vi "TestColletion2.vi"() -> ()   [LabVIEW 2018]
uses:
  <vilib>/Utility/error.llb/whitespace.ctl
panel:
  out "数据处理 2":bool
  out "AI0":bool
  out "AI1":bool
  out "AI2":bool
  out "AI3":bool
  out "AI4":bool
  out "AI5":bool
  out "AI6":bool
  out "AI7":bool
  out "AI8":bool
  out "AI9":bool
  out "AI10":bool
  out "AI11":bool
  out "AI12":bool
  out "AI13":bool
  out "AI14":bool
  out "AI15":bool
  out "数据处理及上传控制":i32
  out "数据1":dbl[](array[numeric])
  out "输出数组1":dbl[](array[numeric])
  out "AI 0 size(s)":i32
  out "数据2":dbl[](array[numeric])
  out "数据3":dbl[](array[numeric])
  out "数据4":dbl[](array[numeric])
  out "数据5":dbl[](array[numeric])
  out "数据6":dbl[](array[numeric])
  out "数据7":dbl[](array[numeric])
  out "数据8":dbl[](array[numeric])
  out "数据9":dbl[](array[numeric])
  out "数据10":dbl[](array[numeric])
  out "数据11":dbl[](array[numeric])
  out "数据12":dbl[](array[numeric])
  out "数据13":dbl[](array[numeric])
  out "数据14":dbl[](array[numeric])
  out "数据15":dbl[](array[numeric])
  out "数据16":dbl[](array[numeric])
  out "输出数组16":dbl[](array[numeric])
  out "输出数组15":dbl[](array[numeric])
  out "输出数组14":dbl[](array[numeric])
  out "输出数组13":dbl[](array[numeric])
  out "输出数组12":dbl[](array[numeric])
  out "输出数组11":dbl[](array[numeric])
  out "输出数组10":dbl[](array[numeric])
  out "输出数组9":dbl[](array[numeric])
  out "输出数组8":dbl[](array[numeric])
  out "输出数组7":dbl[](array[numeric])
  out "输出数组6":dbl[](array[numeric])
  out "输出数组5":dbl[](array[numeric])
  out "输出数组4":dbl[](array[numeric])
  out "输出数组3":dbl[](array[numeric])
  out "输出数组2":dbl[](array[numeric])
  out "大小":i32
  out "数组":string[][](array[string])
  out "数值 3":i32
  out "字符串":string
  out "数值 2":i32
  out "数值":i32
  out "特征值16":string
  out "特征值15":string
  out "特征值14":string
  out "特征值13":string
  out "特征值12":string
  out "特征值11":string
  out "特征值10":string
  out "特征值9":string
  out "特征值8":string
  out "特征值7":string
  out "特征值6":string
  out "特征值5":string
  out "特征值4":string
  out "特征值3":string
  out "特征值2":string
  out "特征值1":string
  in  "XB_NLP2.IClass1":refnum<k7>
  in  "noisy1.IClass1":refnum<k7>
  out "AI 1 size(s)":i32
  in  "输入电压":sgl(ring)=5.0 items=["10"=10, "5"=5]
  out "SQL语句":string
  in  "通道模式":u8(ring)=3 items=["DIFF"=0, "NRSE"=1, "RSE"=3]
  in  "驱动编号":i32
  out "subarray":string[](array[string])
  in  "停止":bool
  out "AI 15 size(s)":i32
  out "AI 14 size(s)":i32
  out "AI 13 size(s)":i32
  out "AI 12 size(s)":i32
  out "AI 11 size(s)":i32
  out "AI 10 size(s)":i32
  out "AI 9 size(s)":i32
  out "AI 8 size(s)":i32
  out "AI 7 size(s)":i32
  out "AI 4 size(s)":i32
  out "AI 5 size(s)":i32
  out "AI 6 size(s)":i32
  out "AI 3 size(s)":i32
  out "AI 2 size(s)":i32
  in  "主选项卡":T1(tab)
  in  "采样次数":u32=5 format="采样次数：%.0f"
  in  "搜索按钮":bool
  in  "间隔时间":i32 format="时间(min)：%.0f"
  in  "sym":string="sym10"
  in  "lev":i32=3 format="lev: %.0f"
  out "数据库状态":errorcluster caption="采集卡状态"
  out "采集卡状态":errorcluster
  in  "暂停":bool
  in  "关闭":bool
  in  "延时":bool
  out "布尔":bool
  in  "数据处理":bool
  in  "初始化":bool
  out "上传到数据库":bool
  in  "数据库":bool
  in  "开始":bool
  in  "主页按钮 8":bool
  in  "主页按钮 9":bool
  out "当前时间":timestamp format="时间：%<%H:%M:%S %x>T"
  in  "查看单传感器采集的数据":bool
  in  "历史查询":bool
  in  "查看当前特征值":bool
  in  "查看当前数据波形":bool
  in  "查看去噪后波形":bool
  in  "创建特征值数据表":bool
  in  "创建原始数据表":bool
  in  "通道选择":bool[](array[boolean])=[TRUE, FALSE, FALSE, FALSE, FALSE, FALSE, FALSE, FALSE, FALSE, FALSE, FALSE, FALSE, FALSE, FALSE, FALSE, FALSE]
  out "过程提示":string
  in  "采样率":u32=1000 format="采样率：%.0f"
  in  "主页按钮 2":bool
  in  "清空传感器数据表":bool
  in  "清空数据":bool
  in  "显示全部数据":bool
  in  "保存16个传感器的数据":bool
  out "全部数据":string[][](table)
  in  "主页按钮":bool
  in  "原始数据选项卡":enum32{"1 - 8", "9 - 16"}(tab)
  out "AI 3 波形":dbl[](graph)
  out "AI 2 波形":dbl[](graph)
  out "AI 1 波形":dbl[](graph)
  out "AI 4 波形":dbl[](graph)
  out "AI 5 波形":dbl[](graph)
  out "AI 7 波形":dbl[](graph)
  out "AI 6 波形":dbl[](graph)
  out "AI 11 波形":dbl[](graph)
  out "AI 8 波形":dbl[](graph)
  out "AI 9 波形":dbl[](graph)
  out "AI 10 波形":dbl[](graph)
  out "AI 12 波形":dbl[](graph)
  out "AI 13 波形":dbl[](graph)
  out "AI 14 波形":dbl[](graph)
  out "AI 15 波形":dbl[](graph)
  in  "主页按钮 3":bool
  in  "去噪波形选项卡":enum32{"1 - 8 ", "9 - 16"}(tab)
  out "AI2去噪后波形图":dbl[][](graph)
  out "AI3去噪后波形图":dbl[][](graph)
  out "AI4去噪后波形图":dbl[][](graph)
  out "AI5去噪后波形图":dbl[][](graph)
  out "AI6去噪后波形图":dbl[][](graph)
  out "AI7去噪后波形图":dbl[][](graph)
  out "AI1去噪后波形图":dbl[][](graph)
  out "AI0去噪后波形图":dbl[][](graph)
  out "AI8去噪后波形图":dbl[][](graph)
  out "AI9去噪后波形图":dbl[][](graph)
  out "AI10去噪后波形图":dbl[][](graph)
  out "AI11去噪后波形图":dbl[][](graph)
  out "AI2去噪后波形图":dbl[][](graph)
  out "AI13去噪后波形图":dbl[][](graph)
  out "AI14去噪后波形图":dbl[][](graph)
  out "AI15去噪后波形图":dbl[][](graph)
  in  "主页按钮 4":bool
  out "AI0特征值":dbl[][](array[numeric])
  out "AI1特征值":dbl[][](array[numeric])
  out "AI3特征值":dbl[][](array[numeric])
  out "AI5特征值":dbl[][](array[numeric])
  out "AI4特征值":dbl[][](array[numeric])
  out "AI2特征值":dbl[][](array[numeric])
  out "AI6特征值":dbl[][](array[numeric])
  out "AI8特征值":dbl[][](array[numeric])
  out "AI10特征值":dbl[][](array[numeric])
  out "AI11特征值":dbl[][](array[numeric])
  out "AI12特征值":dbl[][](array[numeric])
  out "AI13特征值":dbl[][](array[numeric])
  out "AI14特征值":dbl[][](array[numeric])
  out "AI7特征值":dbl[][](array[numeric])
  out "AI9特征值":dbl[][](array[numeric])
  out "AI15特征值":dbl[][](array[numeric])
  in  "主页按钮 5":bool
  in  "历史查询选项卡":enum32{"原始数据查询", "健康值查询"}(tab)
  out "状态提示":string
  out "波形图 2":dbl[](graph)
  out "查询数据":string[][](table)
  in  "文件名":string
  in  "保存地址":path
  in  "保存":bool
  in  "传感器":T2(ring)
  in  "查询":bool
  in  "从":timestamp
  in  "到":timestamp
  in  "传感器":T2(ring)
  in  "到":timestamp
  in  "从":timestamp
  out "健康值查询结果":string[][](table)
  in  "显示健康值":bool
  in  "传感器数据查询":bool
  in  "健康值查询":bool
  in  "主页按钮 6":bool
  out "波形图 3":dbl[](graph)
  out "当前组波形":dbl[](graph)
  in  "主页按钮 7":bool
  out "AI0特征值 2":dbl[][](array[numeric])
  out "去噪后波形图":dbl[][](graph)
  # "包装设备状态监测与预测系统"
  # "请务必将传感器接到采集卡的 AI 0 通道"
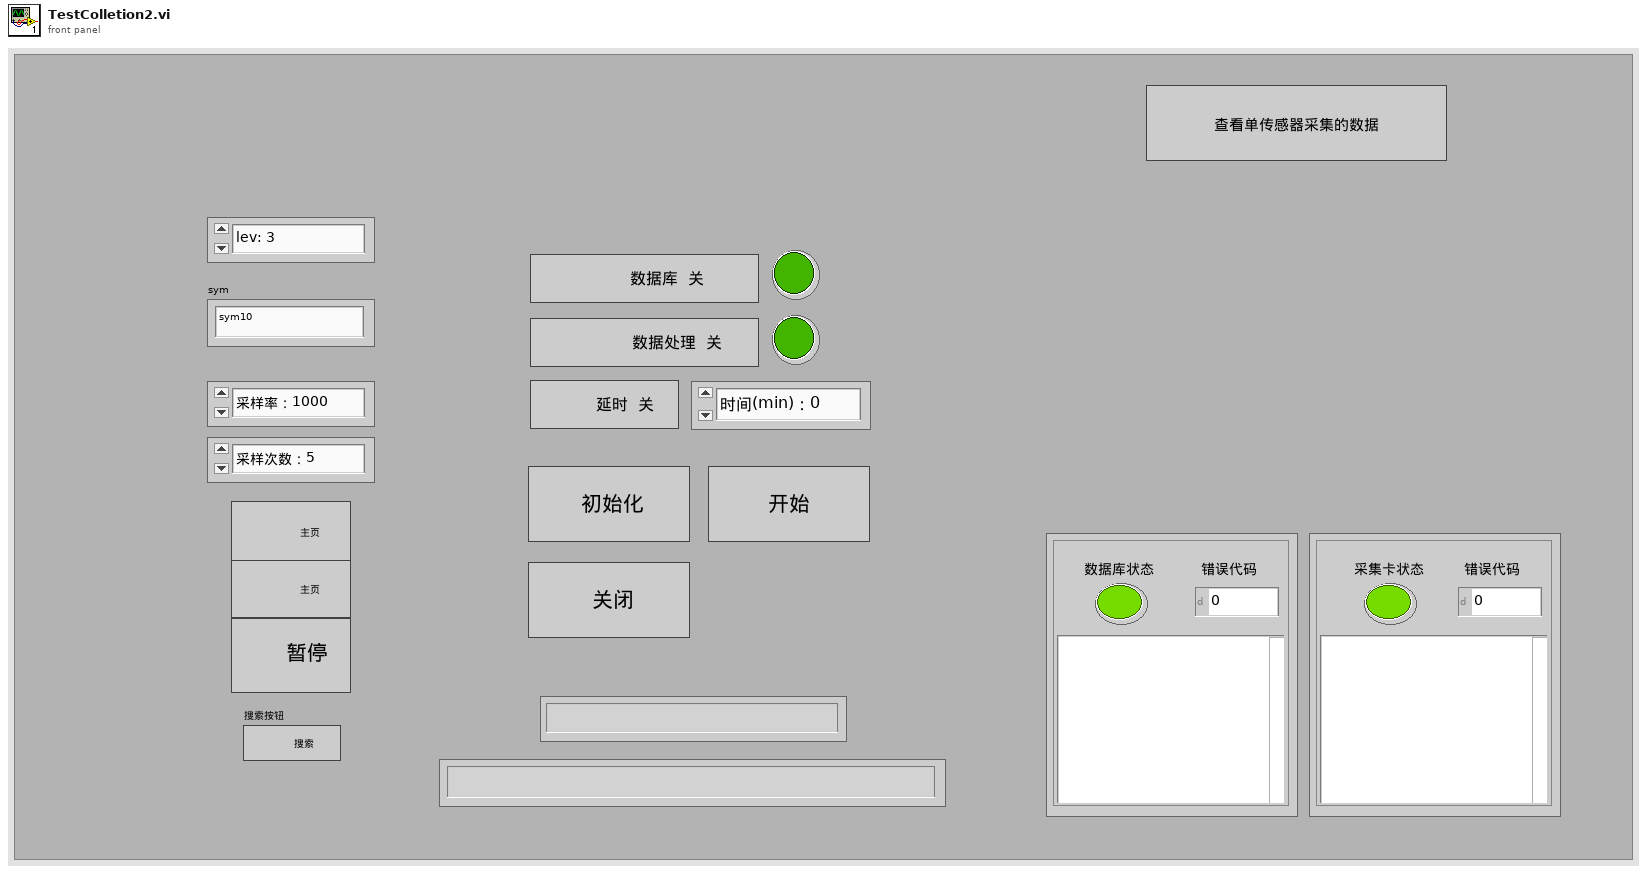
[diagram p1: front panel]
types:
  T1 = enum32{"端口设置", "传感器数据", "原始数据波形", "去噪后的波形", "特征值数据", "健康值记录", "历史查询", "单传感器测试"}
  T2 = enum16{"sensor1", "sensor2", "sensor3", "sensor4", "sensor5", "sensor6", "sensor7", "sensor8", "sensor9", "sensor10", "sensor11", "sensor12", "sensor13", "sensor14", "sensor15", "sensor16"}
  T3 = typedef "whitespace.ctl" = u16
  T4 = enum16{"open", "replace", "create", "open or create", "replace or create", "replace or create with confirmation"}
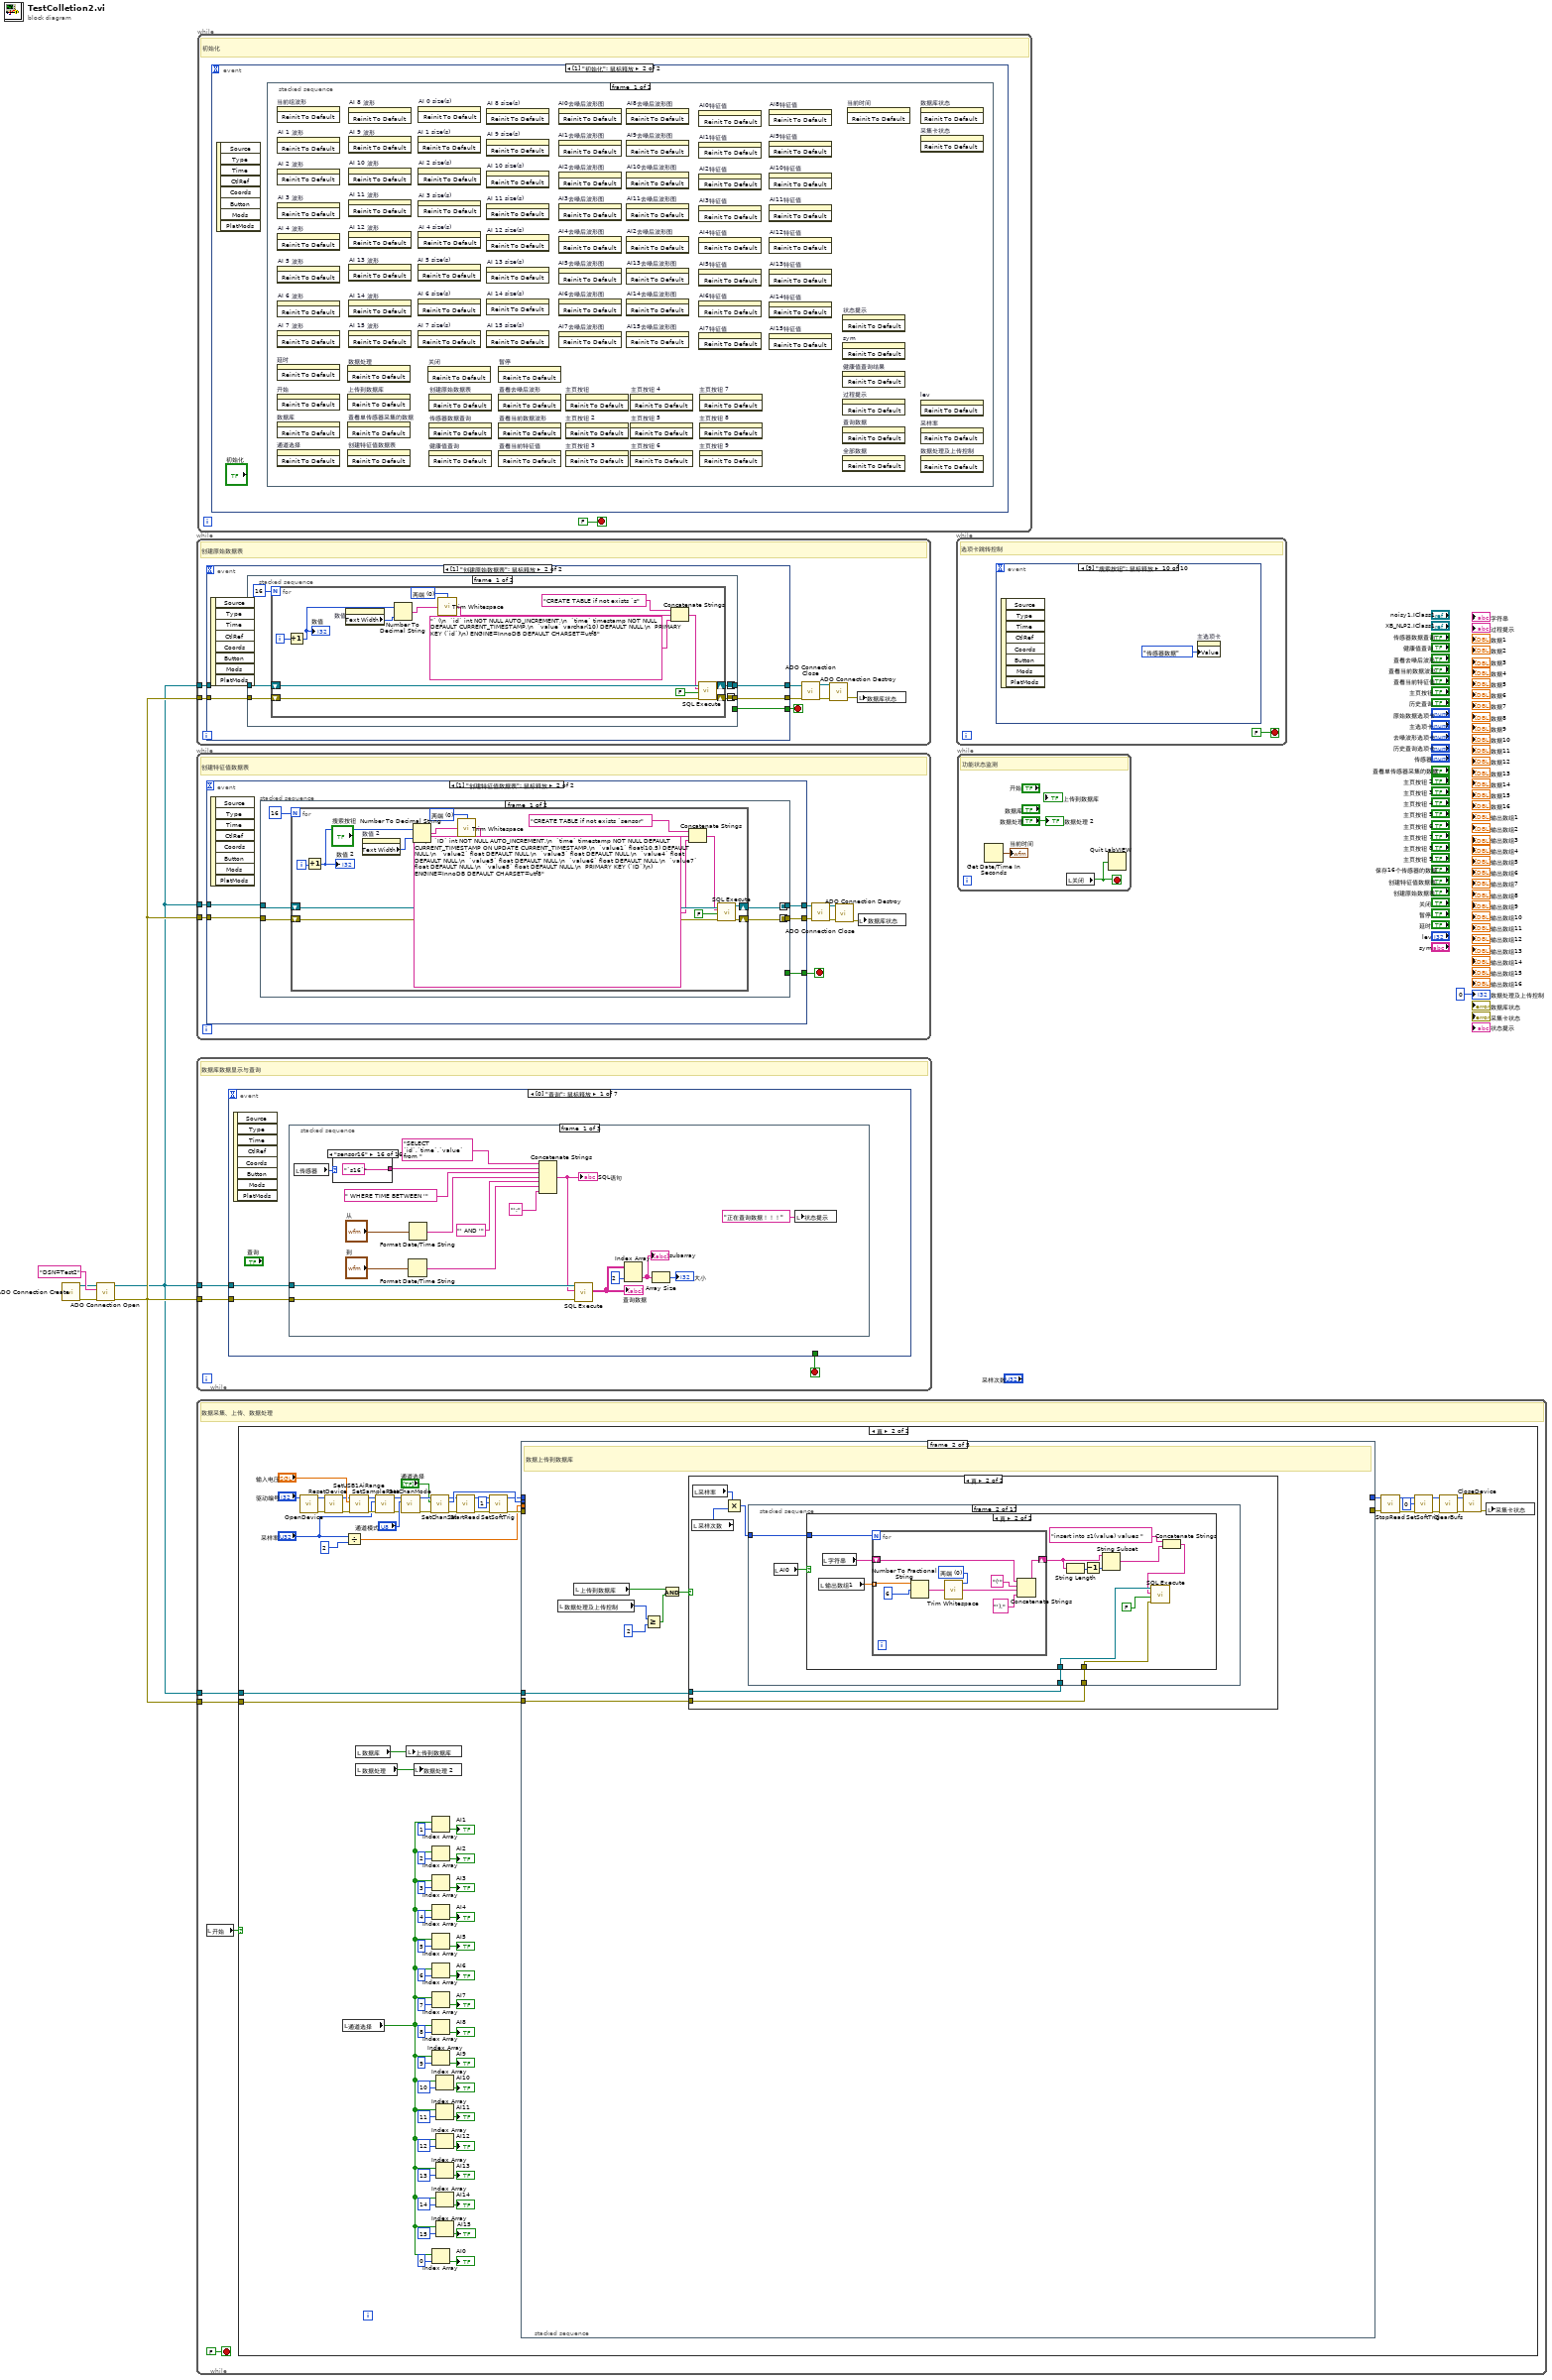
[diagram p0: block diagram]
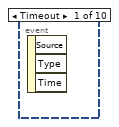
[diagram p2: hidden frame]
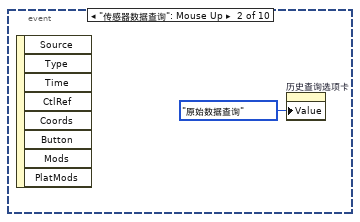
[diagram p3: hidden frame]
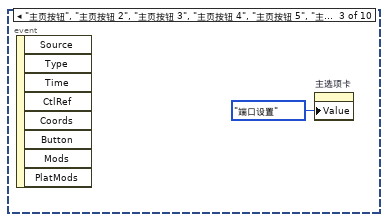
[diagram p4: hidden frame]
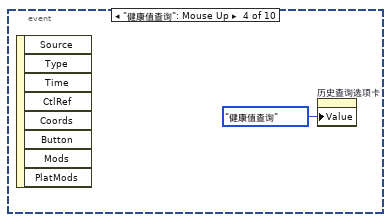
[diagram p5: hidden frame]
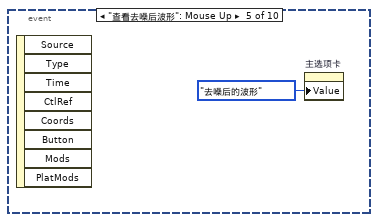
[diagram p6: hidden frame]
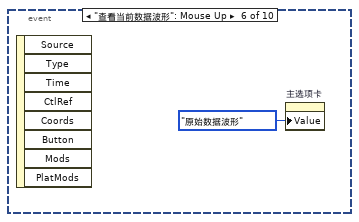
[diagram p7: hidden frame]
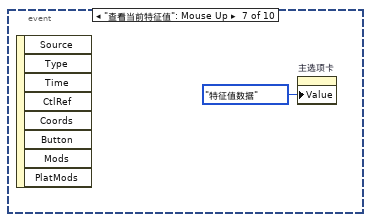
[diagram p8: hidden frame]
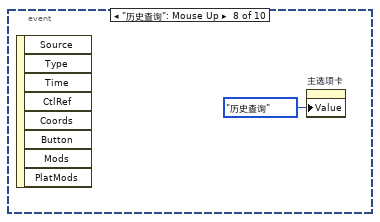
[diagram p9: hidden frame]
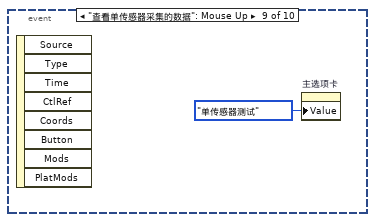
[diagram p10: hidden frame]
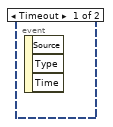
[diagram p11: hidden frame]
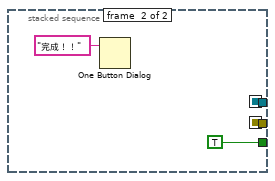
[diagram p12: hidden frame]
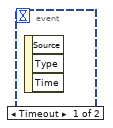
[diagram p13: hidden frame]
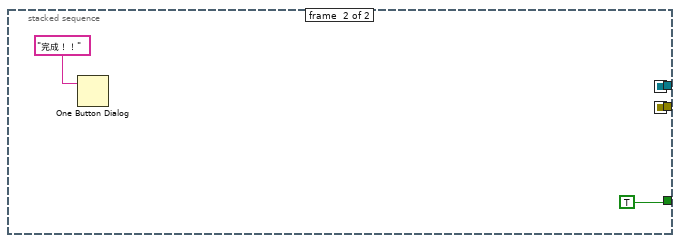
[diagram p14: hidden frame]
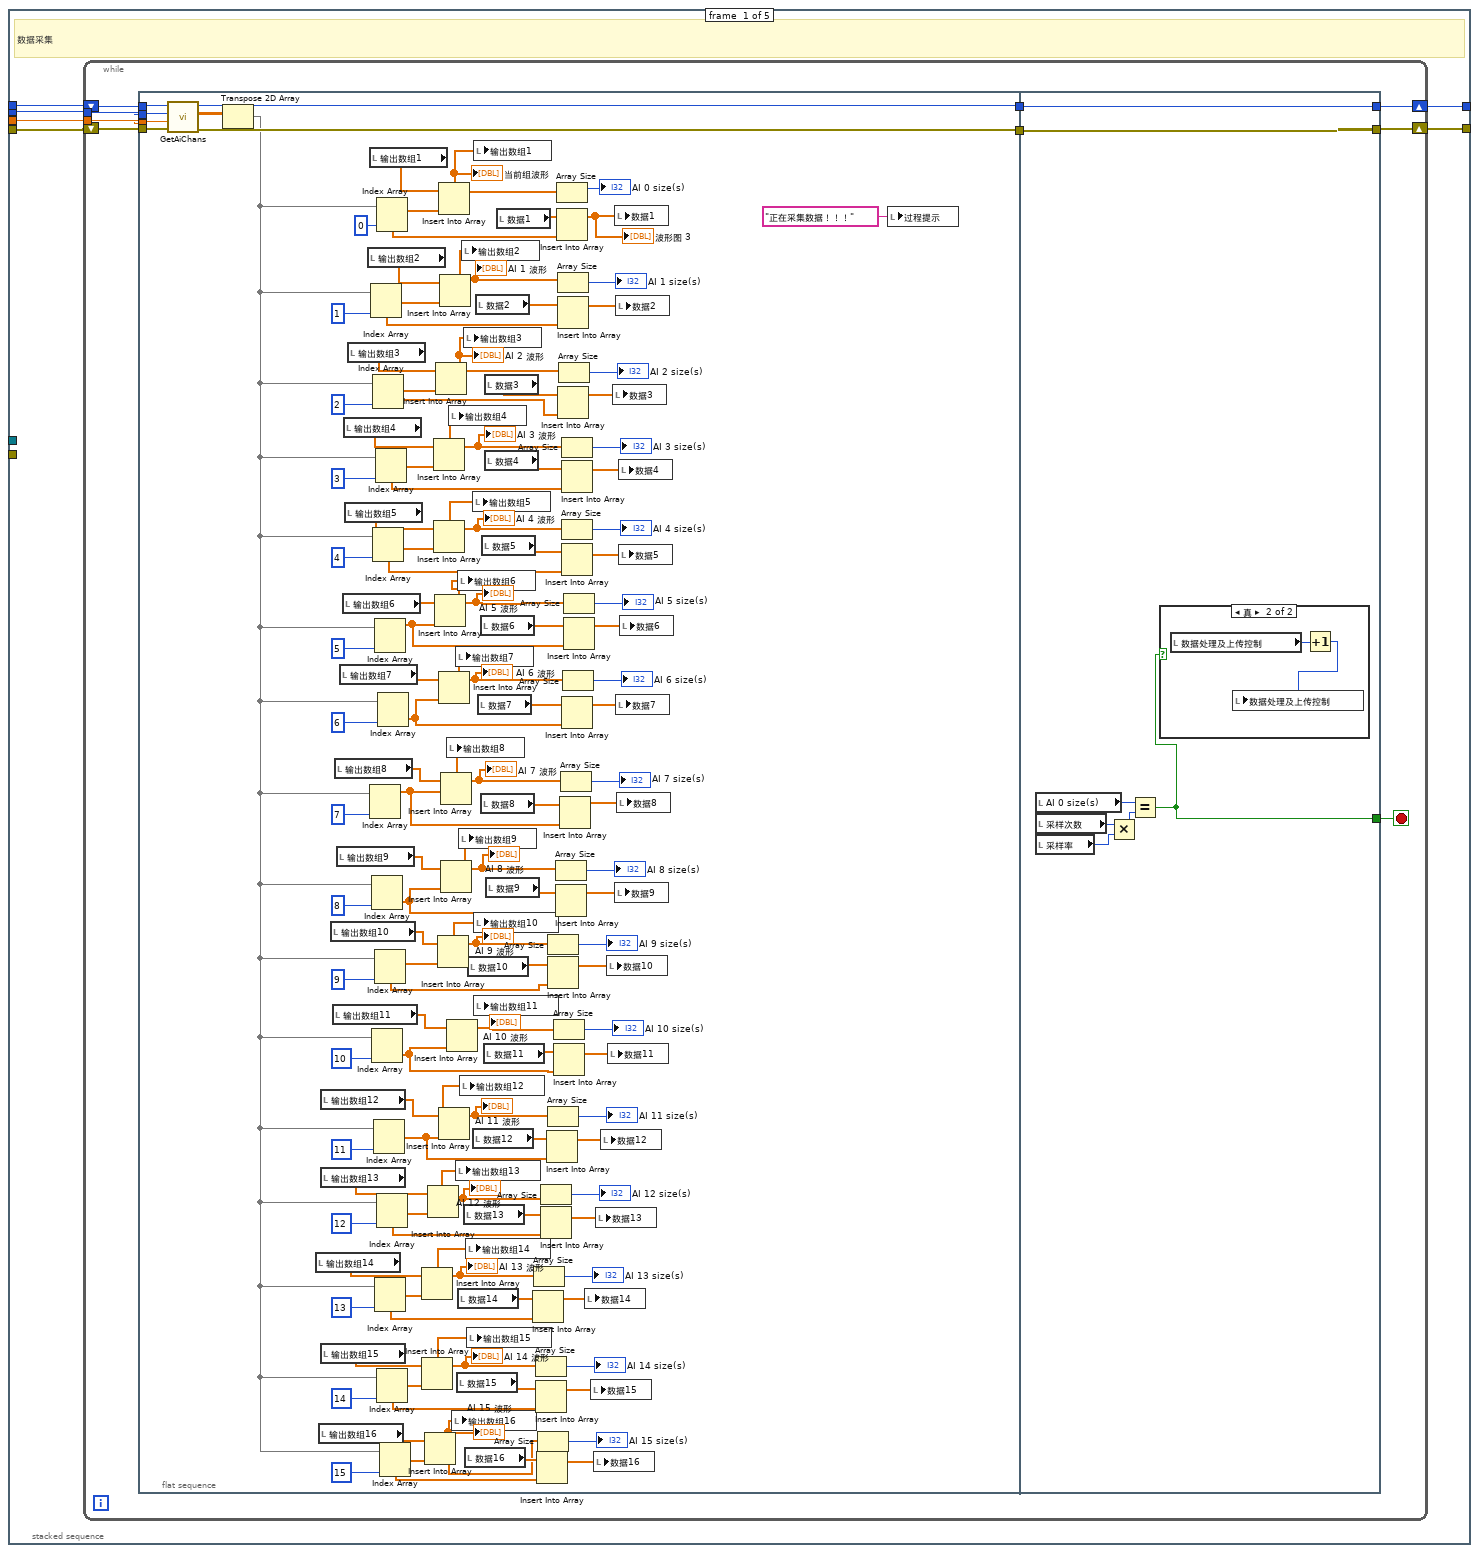
[diagram p16: hidden frame]
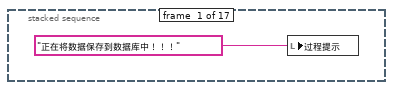
[diagram p19: hidden frame]
diagram:
  n1 = call "ADO Connection Create.vi"() -> ("error out"=w4:errorcluster, "ADODB._Connection Out"=w5:refnum<k7>)  [unwired: 10 in]
  n2 = call "ADO Connection Open.vi"("error in (no error)"=w4, "ConnectionString"="DSN=Test2", "ADODB._Connection In"=w5) -> ("error out"=w3:errorcluster, "ADODB._Connection Out"=w2:refnum<k7>)  [unwired: 7 in]
  n3 = while {
    tunnel: w3 -> [w14]
    tunnel: w2 -> [w13]
    stop <- w8 stop-if-true
    # "创建原始数据表"
    n4 = event shown="[1] \"创建原始数据表\": 鼠标释放" {
      selector: _ -> [_ _]
      dyn-events: _ -> [_ _]
      timeout: _ -> [_ _]
      tunnel: w13 -> [_ w19]
      tunnel: w14 -> [_ w18]
      tunnel: [_ w17] -> w9
      tunnel: [_ w16] -> w10
      tunnel: [_ w15] -> w8
      event Timeout {
        n5 = event-data() -> ()  [unwired: 1 in, 3 out]
      }
      event "创建原始数据表": Mouse Up {
        n6 = event-data() -> ()  [unwired: 1 in, 8 out]
        n7 = stacked-sequence {
          seq-local: [w22 _] -> [_ w42]
          seq-local: [w21 _] -> [_ w41]
          tunnel: w19 -> [w24 _]
          tunnel: w18 -> [w23 _]
          tunnel: [_ w42] -> w17
          tunnel: [_ w41] -> w16
          tunnel: [_ TRUE] -> w15
          frame #0 {
            n8 = for {
              N: 16 -> [_]
              shift-right: [w34] -> w21
              shift-left: w24 -> [w38]
              shift-right: [w35] -> w22
              shift-left: w23 -> [w37]
              i -> [w26]
              w28 = T3 0 items=["两端", "字符串首端", "字符串末端"] ("location (both)")
              n9 = Increment(x=w26) -> (x+1=w25:i32)
              "数值" <- w25
              n10 = property on="数值" class="DigNum (严格)"() -> ("Text Width"=w27:u32)  [unwired: 2 in, 2 out]
              n11 = Number To Decimal String(number=w25, width (-)=w27) -> (decimal integer string=w30:string)
              n12 = call <vilib>:"Trim Whitespace.vi"("string"=w30, "location (both)"=w28) -> ("trimmed string"=w29:string)
              n13 = Concatenate Strings("CREATE TABLE if not exists `s", w29, "` (\n  `id` int NOT NULL AUTO_INCREMENT,\n  `time` timestamp NOT NULL DEFAULT CURRENT_TIMESTAMP,\n  `value` varchar(10) DEFAULT NULL,\n  PRIMARY KEY (`id`)\n) ENGINE=InnoDB DEFAULT CHARSET=utf8") -> (w31:string)
              n14 = call "SQL Execute.vi"("error in (no error)"=w37, "Return Data (T)"=FALSE, "Command Text"=w31, "ADODB._Connection In"=w38) -> ("error out"=w35:errorcluster, "ADODB._Connection Out"=w34:refnum<k7>)  [unwired: 4 in, 2 out]
            }
          }
          frame #1 {
            n15 = One Button Dialog(message="完成！！" ("消息")) -> ()  [unwired: 1 in, 1 out]
          }
        }
      }
    }
    n16 = call "ADO Connection Close.vi"("error in (no error)"=w9, "ADODB._Connection In"=w10) -> ("error out"=w11:errorcluster, "ADODB._Connection Out"=w12:refnum<k7>)  [unwired: 8 in]
    n17 = call "ADO Connection Destroy.vi"("error in (no error)"=w11, "ADODB._Connection In"=w12) -> ("error out"=w7:errorcluster)  [unwired: 9 in]
    n18 = local write "数据库状态"(w7) -> ()
  }
  n19 = while {
    tunnel: w3 -> [w50]
    tunnel: w2 -> [w49]
    stop <- w44 stop-if-true
    # "创建特征值数据表"
    n20 = event shown="[1] \"创建特征值数据表\": 鼠标释放" {
      selector: _ -> [_ _]
      dyn-events: _ -> [_ _]
      timeout: _ -> [_ _]
      tunnel: w49 -> [_ w55]
      tunnel: w50 -> [_ w54]
      tunnel: [_ w53] -> w45
      tunnel: [_ w52] -> w46
      tunnel: [_ w51] -> w44
      event Timeout {
        n21 = event-data() -> ()  [unwired: 1 in, 3 out]
      }
      event "创建特征值数据表": Mouse Up {
        n22 = event-data() -> ()  [unwired: 1 in, 8 out]
        n23 = stacked-sequence {
          seq-local: [w57 _] -> [_ w78]
          seq-local: [w56 _] -> [_ w77]
          tunnel: w55 -> [w59 _]
          tunnel: w54 -> [w58 _]
          tunnel: [_ w78] -> w53
          tunnel: [_ w77] -> w52
          tunnel: [_ TRUE] -> w51
          frame #0 {
            n24 = for {
              N: 16 -> [_]
              shift-right: [w70] -> w57
              shift-left: w59 -> [w74]
              shift-right: [w71] -> w56
              shift-left: w58 -> [w73]
              i -> [w62]
              w64 = T3 0 items=["两端", "字符串首端", "字符串末端"] ("location (both)")
              n25 = Increment(x=w62) -> (x+1=w61:i32)
              "数值 2" <- w61
              n26 = property on="数值 2" class="DigNum (严格)"() -> ("Text Width"=w63:u32)  [unwired: 2 in, 2 out]
              n27 = Number To Decimal String(number=w61, width (-)=w63) -> (decimal integer string=w66:string)
              n28 = call <vilib>:"Trim Whitespace.vi"("string"=w66, "location (both)"=w64) -> ("trimmed string"=w65:string)
              n29 = Concatenate Strings("CREATE TABLE if not exists `sensor", w65, "` (\n  `ID` int NOT NULL AUTO_INCREMENT,\n  `time` timestamp NOT NULL DEFAULT CURRENT_TIMESTAMP ON UPDATE CURRENT_TIMESTAMP,\n  `value1` float(10,5) DEFAULT NULL,\n  `value2` float DEFAULT NULL,\n  `value3` float DEFAULT NULL,\n  `value4` float DEFAULT NULL,\n  `value5` float DEFAULT NULL,\n  `value6` float DEFAULT NULL,\n  `value7` float DEFAULT NULL,\n  `value8` float DEFAULT NULL,\n  PRIMARY KEY (`ID`)\n) ENGINE=InnoDB DEFAULT CHARSET=utf8") -> (w67:string)
              n30 = call "SQL Execute.vi"("error in (no error)"=w73, "Return Data (T)"=FALSE, "Command Text"=w67, "ADODB._Connection In"=w74) -> ("error out"=w71:errorcluster, "ADODB._Connection Out"=w70:refnum<k7>)  [unwired: 4 in, 2 out]
            }
          }
          frame #1 {
            n31 = One Button Dialog(message="完成！！" ("消息")) -> ()  [unwired: 1 in, 1 out]
          }
        }
      }
    }
    n32 = call "ADO Connection Close.vi"("error in (no error)"=w46, "ADODB._Connection In"=w45) -> ("error out"=w47:errorcluster, "ADODB._Connection Out"=w48:refnum<k7>)  [unwired: 8 in]
    n33 = call "ADO Connection Destroy.vi"("error in (no error)"=w47, "ADODB._Connection In"=w48) -> ("error out"=w43:errorcluster)  [unwired: 9 in]
    n34 = local write "数据库状态"(w43) -> ()
  }
  n35 = while {
    tunnel: w3 -> [w81]
    tunnel: w2 -> [w80]
    stop <- w79 stop-if-true
    # "数据库数据显示与查询"
    n36 = event shown="[0] \"查询\": 鼠标释放" {
      selector: _ -> [_ _ _ _ _ _ _]
      dyn-events: _ -> [_ _ _ _ _ _ _]
      timeout: _ -> [_ _ _ _ _ _ _]
      tunnel: w81 -> [w82 _ _ w151 w172 w191 _]
      tunnel: w80 -> [w83 _ _ w152 w173 w190 _]
      tunnel: [_ _ TRUE _ _ _ _] -> w79
      event "查询": Mouse Up {
        n37 = event-data() -> ()  [unwired: 1 in, 8 out]
        n38 = stacked-sequence {
          tunnel: w83 -> [w101 _ _]
          tunnel: w82 -> [w100 _ _]
          frame #0 {
            n39 = local read "传感器"() -> (w91:T2)
            n40 = case shown="\"sensor16\"" w91 {
              tunnel: ["`s1`" "`s2`" "`s3`" "`s4`" "`s5`" "`s6`" "`s7`" "`s8`" "`s9`" "`s10`" "`s11`" "`s12`" "`s13`" "`s14`" "`s15`" "`s16`"] -> w86
              frame "sensor1", Default {
              }
              frame "sensor2" {
              }
              frame "sensor3" {
              }
              frame "sensor4" {
              }
              frame "sensor5" {
              }
              frame "sensor6" {
              }
              frame "sensor7" {
              }
              frame "sensor8" {
              }
              frame "sensor9" {
              }
              frame "sensor10" {
              }
              frame "sensor11" {
              }
              frame "sensor12" {
              }
              frame "sensor13" {
              }
              frame "sensor14" {
              }
              frame "sensor15" {
              }
              frame "sensor16" {
              }
            }
            n41 = Format Date/Time String(seconds (now)="到") -> (date/time string=w94:string)  [unwired: 2 in]
            n42 = Format Date/Time String(seconds (now)="从") -> (date/time string=w93:string)  [unwired: 2 in]
            n43 = Concatenate Strings("SELECT `id`,`time`,`value` from " ("string"), w86, " WHERE TIME BETWEEN '" ("string"), w93, "' AND '" ("string"), w94, "';" ("string")) -> (w97:string)
            "SQL语句" <- w97
            n44 = call "SQL Execute.vi"("error in (no error)"=w100, "Command Text"=w97, "ADODB._Connection In"=w101) -> ("Data"=w88:string[][])  [unwired: 5 in, 3 out]
            "查询数据" <- w88
            n45 = Index Array(array=w88, index (col)=2 ("disabled index (col)")) -> (element=w89:string[])  [unwired: 1 in]
            "subarray" <- w89
            n46 = Array Size(array=w89) -> (size(s)=→"大小":i32)
            n47 = local write "状态提示"("正在查询数据！！！" ("状态提示")) -> ()
          }
          frame #1 {
            n48 = local read "大小"() -> (w120:i32)
            n49 = for {
              N: w120 -> [_]
              shift-right: [w122] -> w119
              shift-left: dbl[] [] -> [w123]
              i -> [w125]
              n50 = local read "subarray"() -> (w126:string[])
              n51 = Index Array(array=w126, index=w125) -> (element=w128:string)
              n52 = Fract/Exp String To Number(string=w128) -> (number=w127:dbl)  [unwired: 3 in, 1 out]
              n53 = Build Array(w127) -> (w124:dbl[])
              n54 = Insert Into Array(array=w123, index=w125, new element=w124) -> (w122:dbl[])
            }
            "波形图 2" <- w119
            n55 = local write "状态提示"("正在绘制波形" ("状态提示")) -> ()
          }
          frame #2 {
            n56 = One Button Dialog(message="查询及绘图完成！！！" ("消息")) -> ()  [unwired: 1 in, 1 out]
          }
        }
      }
      event "保存": Mouse Up {
        n57 = event-data() -> ()  [unwired: 1 in, 8 out]
        n58 = flat-sequence {
          frame #0 {
            n59 = property on="查询数据" class="Tbl (严格)"() -> ("Value"=w137:string[][])  [unwired: 2 in, 2 out]
            n60 = Index Array(array=w137, index (col)=2 ("disabled index (col)")) -> (element=w135:string[])  [unwired: 1 in]
            n61 = Concatenate Strings("文件名", ".csv" ("name or relative path")) -> (w141:string)
            n62 = Build Path(base path="保存地址", name or relative path=w141) -> (appended path=w142:path)
            n63 = Array To Spreadsheet String(delimiter (Tab)="\r\n", array=w135, 3:"" ("format string")) -> (spreadsheet string=w132:string)
            n64 = Open/Create/Replace File(file path (use dialog)=w142, operation (0:open)=T4."replace or create", access (0:read/write)=enum16{"read/write", "read-only", "write-only"}."read/write") -> (refnum out=w146:refnum<file>, error out=w147:errorcluster)  [unwired: 3 in, 1 out]
            n65 = Write to Binary File(file (use dialog)=w146, data=w132, error in=w147) -> (refnum out=w144:refnum<file>, error out=w145:errorcluster)  [unwired: 3 in, 1 out]
            n66 = Close File(refnum=w144, error in=w145) -> (error out=w143:errorcluster)  [unwired: 1 out]
            n67 = call <vilib>:"Simple Error Handler.vi"("error in (no error)"=w143) -> ()  [unwired: 4 in, 5 out]
          }
          frame #1 {
            n68 = One Button Dialog(message="数据保存完成！！！" ("消息")) -> ()  [unwired: 1 in, 1 out]
          }
        }
      }
      event "停止": Mouse Up {
        n69 = event-data() -> ()  [unwired: 1 in, 8 out]
      }
      event "显示全部数据": Mouse Up {
        n70 = event-data() -> ()  [unwired: 1 in, 8 out]
        n71 = for {
          N: 16 -> [_]
          tunnel: w152 -> [w169]
          tunnel: w151 -> [w168]
          i -> [w154]
          w162 = T3 0 items=["两端", "字符串首端", "字符串末端"] ("location (both)")
          n72 = Increment(x=w154) -> (x+1=w153:i32)
          "数值 3" <- w153
          n73 = property on="数值 3" class="DigNum (严格)"() -> ("Text Width"=w165:u32)  [unwired: 2 in, 2 out]
          n74 = Number To Fractional String(number=w153, width (-)=w165) -> (F-format string=w163:string)  [unwired: 2 in]
          n75 = call <vilib>:"Trim Whitespace.vi"("string"=w163, "location (both)"=w162) -> ("trimmed string"=w161:string)
          n76 = Concatenate Strings("select `value` from `s;" ("string"), w161, "`;") -> (w159:string)
          n77 = call "SQL Execute.vi"("error in (no error)"=w168, "Return Data (T)"=FALSE, "Command Text"=w159, "ADODB._Connection In"=w169) -> ("Data"=w167:string[][])  [unwired: 4 in, 3 out]
          n78 = Index Array(array=w167, index (col)=0 ("禁用的索引 (列)")) -> (element=w157:string[])  [unwired: 1 in]
          n79 = local read "数组"() -> (w158:string[][])
          n80 = Insert Into Array(array=w158, index (row)=w153, new element=w157) -> (→"全部数据":string[][])  [unwired: 1 in]
        }
      }
      event "显示健康值": Mouse Up {
        n81 = event-data() -> ()  [unwired: 1 in, 8 out]
        n82 = case shown="\"sensor16\"" "传感器" {
          tunnel: ["`s1`" "`s2`" "`s3`" "`s4`" "`s5`" "`s6`" "`s7`" "`s8`" "`s9`" "`s10`" "`s11`" "`s12`" "`s13`" "`s14`" "`s15`" "`s16`"] -> _
          frame "sensor1", Default {
          }
          frame "sensor2" {
          }
          frame "sensor3" {
          }
          frame "sensor4" {
          }
          frame "sensor5" {
          }
          frame "sensor6" {
          }
          frame "sensor7" {
          }
          frame "sensor8" {
          }
          frame "sensor9" {
          }
          frame "sensor10" {
          }
          frame "sensor11" {
          }
          frame "sensor12" {
          }
          frame "sensor13" {
          }
          frame "sensor14" {
          }
          frame "sensor15" {
          }
          frame "sensor16" {
          }
        }
        n83 = call "SQL Execute.vi"("error in (no error)"=w172, "Command Text"="", "ADODB._Connection In"=w173) -> ()  [unwired: 5 in, 4 out]
      }
      event "清空数据": Mouse Up {
        # "清空数据库的全部数据"
        n84 = event-data() -> ()  [unwired: 1 in, 8 out]
        n85 = call "SQL Execute.vi"("error in (no error)"=w191, "Return Data (T)"=FALSE, "Command Text"="truncate s1;" ("string"), "ADODB._Connection In"=w190) -> ()  [unwired: 4 in, 4 out]
        n86 = One Button Dialog(message="数据已全部清除", button name ("OK")="确定     ") -> ()  [unwired: 1 out]
      }
      event "清空传感器数据表": Mouse Up {
        n87 = event-data() -> ()  [unwired: 1 in, 8 out]
        n88 = flat-sequence {
          frame #0 {
            n89 = invoke on="全部数据" class="Tbl (strict)" method="Reinit To Default"() -> ()  [unwired: 3 in, 3 out]
          }
          frame #1 {
            n90 = One Button Dialog(message="清空完毕！！！" ("消息")) -> ()  [unwired: 1 in, 1 out]
          }
        }
      }
    }
  }
  n91 = while {
    tunnel: w3 -> [w197]
    tunnel: w2 -> [w198]
    stop <- FALSE stop-if-true
    # "数据采集、上传、数据处理"
    n92 = local read "开始"() -> (w199:bool)
    n93 = case shown="真" w199 {
      tunnel: w198 -> [_ w262]
      tunnel: w197 -> [_ w261]
      frame False {
      }
      frame True {
        n94 = call "OpenDevice.vi"("DevIndex"="驱动编号") -> ("错误输出"=w244:errorcluster, "DevIndex Output"=w245:i32)  [unwired: 9 in]
        n95 = call "ResetDevice.vi"("错误输入（无错误）"=w244, "DevIndex"=w245) -> ("错误输出"=w247:errorcluster, "DevIndex Output"=w248:i32)  [unwired: 8 in]
        n96 = local read "通道选择"() -> (w203:bool[])
        n97 = Divide(x="采样率", y=u32 2) -> (x/y=w207:dbl)
        n98 = call "SetUSB1AiRange.vi"("错误输入（无错误）"=w247, "Range"="输入电压", "DevIndex"=w248) -> ("错误输出"=w250:errorcluster, "DevIndex Output"=w251:i32)  [unwired: 7 in]
        n99 = local read "数据库"() -> (w205:bool)
        n100 = local read "数据处理"() -> (w206:bool)
        n101 = call "SetSampleRate.vi"("错误输入（无错误）"=w250, "SampleRate"="采样率", "DevIndex"=w251) -> ("错误输出"=w252:errorcluster, "DevIndex Output"=w253:i32)  [unwired: 7 in]
        n102 = call "SetChanMode.vi"("错误输入（无错误）"=w252, "ChanMode"="通道模式", "DevIndex"=w253) -> ("错误输出"=w255:errorcluster, "DevIndex Output"=w256:i32)  [unwired: 7 in]
        n103 = local write "上传到数据库"(w205) -> ()
        n104 = local write "数据处理 2"(w206) -> ()
        n105 = call "SetChanSel.vi"("错误输入（无错误）"=w255, "ChanSel"="通道选择", "DevIndex"=w256) -> ("错误输出"=w260:errorcluster, "ChanSel"=w264:u16, "DevIndex Output"=w259:i32)  [unwired: 6 in]
        n106 = Index Array(array=w203, index=1) -> (element=→"AI1":bool)
        n107 = Index Array(array=w203, index=2) -> (element=→"AI2":bool)
        n108 = Index Array(array=w203, index=3) -> (element=→"AI3":bool)
        n109 = Index Array(array=w203, index=4) -> (element=→"AI4":bool)
        n110 = Index Array(array=w203, index=5) -> (element=→"AI5":bool)
        n111 = Index Array(array=w203, index=6) -> (element=→"AI6":bool)
        n112 = Index Array(array=w203, index=7) -> (element=→"AI7":bool)
        n113 = Index Array(array=w203, index=8) -> (element=→"AI8":bool)
        n114 = Index Array(array=w203, index=9) -> (element=→"AI9":bool)
        n115 = Index Array(array=w203, index=0) -> (element=→"AI0":bool)
        n116 = Index Array(array=w203, index=10) -> (element=→"AI10":bool)
        n117 = Index Array(array=w203, index=11) -> (element=→"AI11":bool)
        n118 = Index Array(array=w203, index=12) -> (element=→"AI12":bool)
        n119 = Index Array(array=w203, index=13) -> (element=→"AI13":bool)
        n120 = Index Array(array=w203, index=14) -> (element=→"AI14":bool)
        n121 = Index Array(array=w203, index=15) -> (element=→"AI15":bool)
        n122 = call "StartRead.vi"("错误输入（无错误）"=w260, "DevIndex"=w259) -> ("错误输出"=w257:errorcluster, "DevIndex Output"=w258:i32)  [unwired: 8 in]
        n123 = call "SetSoftTrig.vi"("错误输入（无错误）"=w257, "Trig"=u8 1, "DevIndex"=w258) -> ("错误输出"=w265:errorcluster, "DevIndex Output"=w263:i32)  [unwired: 7 in]
        n124 = stacked-sequence {
          tunnel: w262 -> [_ w424 w837 _ _]
          tunnel: w261 -> [_ w423 w836 _ _]
          tunnel: w265 -> [w275 _ _ _ _]
          tunnel: w207 -> [w276 _ _ _ _]
          tunnel: w264 -> [w277 _ _ _ _]
          tunnel: w263 -> [w278 _ _ _ _]
          tunnel: [w274 _ _ _ _] -> w242
          tunnel: [w273 _ _ _ _] -> w241
          frame #0 {
            # "数据采集"
            n125 = while {
              tunnel: w277 -> [w286]
              tunnel: w276 -> [w280]
              shift-right: [w285] -> w274
              shift-left: w278 -> [w287]
              shift-right: [w284] -> w273
              shift-left: w275 -> [w279]
              stop <- w281 stop-if-true
              n126 = flat-sequence {
                tunnel: w287 -> [w361]
                tunnel: w286 -> [w360]
                tunnel: w280 -> [w359]
                tunnel: w279 -> [w357]
                tunnel: [w356] -> w283
                tunnel: [w355] -> w282
                tunnel: [w414] -> w284
                tunnel: [w415] -> w285
                tunnel: w283 -> [w415]
                tunnel: w282 -> [w414]
                tunnel: [w412] -> w281
                frame #0 {
                  n127 = call "GetAiChans.vi"("错误输入（无错误）"=w357, "Num"=w359, "ChanSel"=w360, "DevIndex"=w361) -> ("错误输出"=w355:errorcluster, "Ai"=w358:sgl[][], "DevIndex Output"=w356:i32)  [unwired: 4 in, 1 out]
                  n128 = Transpose 2D Array(2D array=w358) -> (transposed array=w288:sgl[][])
                  n129 = local read "输出数组14"() -> (w364:dbl[])
                  n130 = local read "输出数组16"() -> (w362:dbl[])
                  n131 = local read "输出数组12"() -> (w366:dbl[])
                  n132 = local read "输出数组13"() -> (w365:dbl[])
                  n133 = local read "输出数组15"() -> (w363:dbl[])
                  n134 = local read "输出数组10"() -> (w368:dbl[])
                  n135 = local read "输出数组11"() -> (w367:dbl[])
                  n136 = local read "输出数组8"() -> (w370:dbl[])
                  n137 = local read "输出数组9"() -> (w369:dbl[])
                  n138 = local read "输出数组7"() -> (w371:dbl[])
                  n139 = local read "输出数组6"() -> (w372:dbl[])
                  n140 = local read "输出数组4"() -> (w374:dbl[])
                  n141 = local read "输出数组5"() -> (w373:dbl[])
                  n142 = local read "输出数组3"() -> (w375:dbl[])
                  n143 = local read "输出数组2"() -> (w376:dbl[])
                  n144 = local read "输出数组1"() -> (w377:dbl[])
                  n145 = Index Array(array=w288, index (col)=7 ("disabled index (col)")) -> (element=w334:sgl[])  [unwired: 1 in]
                  n146 = Index Array(array=w288, index (col)=1 ("disabled index (col)")) -> (element=w352:sgl[])  [unwired: 1 in]
                  n147 = Index Array(array=w288, index (col)=8 ("disabled index (col)")) -> (element=w331:sgl[])  [unwired: 1 in]
                  n148 = Index Array(array=w288, index (col)=10 ("disabled index (col)")) -> (element=w325:sgl[])  [unwired: 1 in]
                  n149 = Index Array(array=w288, index (col)=2 ("disabled index (col)")) -> (element=w349:sgl[])  [unwired: 1 in]
                  n150 = Index Array(array=w288, index (col)=4 ("disabled index (col)")) -> (element=w343:sgl[])  [unwired: 1 in]
                  n151 = Index Array(array=w288, index (col)=11 ("disabled index (col)")) -> (element=w322:sgl[])  [unwired: 1 in]
                  n152 = Index Array(array=w288, index (col)=5 ("disabled index (col)")) -> (element=w340:sgl[])  [unwired: 1 in]
                  n153 = Index Array(array=w288, index (col)=9 ("disabled index (col)")) -> (element=w328:sgl[])  [unwired: 1 in]
                  n154 = Index Array(array=w288, index (col)=13 ("disabled index (col)")) -> (element=w315:sgl[])  [unwired: 1 in]
                  n155 = Index Array(array=w288, index (col)=3 ("disabled index (col)")) -> (element=w346:sgl[])  [unwired: 1 in]
                  n156 = Index Array(array=w288, index (col)=0 ("index (row)")) -> (element=w354:sgl[])  [unwired: 1 in]
                  n157 = Index Array(array=w288, index (col)=12 ("disabled index (col)")) -> (element=w319:sgl[])  [unwired: 1 in]
                  n158 = Index Array(array=w288, index (col)=14 ("disabled index (col)")) -> (element=w313:sgl[])  [unwired: 1 in]
                  n159 = Index Array(array=w288, index (col)=6 ("disabled index (col)")) -> (element=w337:sgl[])  [unwired: 1 in]
                  n160 = Index Array(array=w288, index (col)=15 ("disabled index (col)")) -> (element=w309:sgl[])  [unwired: 1 in]
                  n161 = Insert Into Array(array=w364, new element=w315) -> (w291:dbl[])  [unwired: 1 in]
                  "AI 13 波形" <- w291
                  n162 = Insert Into Array(array=w363, new element=w313) -> (w290:dbl[])  [unwired: 1 in]
                  "AI 14 波形" <- w290
                  n163 = Insert Into Array(array=w362, new element=w309) -> (w289:dbl[])  [unwired: 1 in]
                  "AI 15 波形" <- w289
                  n164 = Insert Into Array(array=w365, new element=w319) -> (w292:dbl[])  [unwired: 1 in]
                  "AI 12 波形" <- w292
                  n165 = Insert Into Array(array=w374, new element=w346) -> (w301:dbl[])  [unwired: 1 in]
                  "AI 3 波形" <- w301
                  n166 = Insert Into Array(array=w373, new element=w343) -> (w300:dbl[])  [unwired: 1 in]
                  "AI 4 波形" <- w300
                  n167 = Insert Into Array(array=w372, new element=w340) -> (w299:dbl[])  [unwired: 1 in]
                  "AI 5 波形" <- w299
                  n168 = Insert Into Array(array=w375, new element=w349) -> (w302:dbl[])  [unwired: 1 in]
                  "AI 2 波形" <- w302
                  n169 = Insert Into Array(array=w368, new element=w328) -> (w295:dbl[])  [unwired: 1 in]
                  "AI 9 波形" <- w295
                  n170 = Insert Into Array(array=w377, new element=w354) -> (w306:dbl[])  [unwired: 1 in]
                  "当前组波形" <- w306
                  n171 = Insert Into Array(array=w371, new element=w337) -> (w297:dbl[])  [unwired: 1 in]
                  "AI 6 波形" <- w297
                  n172 = Insert Into Array(array=w366, new element=w322) -> (w293:dbl[])  [unwired: 1 in]
                  "AI 11 波形" <- w293
                  n173 = Insert Into Array(array=w376, new element=w352) -> (w303:dbl[])  [unwired: 1 in]
                  "AI 1 波形" <- w303
                  n174 = Insert Into Array(array=w370, new element=w334) -> (w298:dbl[])  [unwired: 1 in]
                  "AI 7 波形" <- w298
                  n175 = Insert Into Array(array=w369, new element=w331) -> (w296:dbl[])  [unwired: 1 in]
                  "AI 8 波形" <- w296
                  n176 = local write "输出数组8"(w298) -> ()
                  n177 = Insert Into Array(array=w367, new element=w325) -> (w294:dbl[])  [unwired: 1 in]
                  "AI 10 波形" <- w294
                  n178 = local write "输出数组4"(w301) -> ()
                  n179 = local write "输出数组16"(w289) -> ()
                  n180 = local write "输出数组7"(w297) -> ()
                  n181 = local write "输出数组13"(w292) -> ()
                  n182 = local read "数据15"() -> (w312:dbl[])
                  n183 = local write "输出数组6"(w299) -> ()
                  n184 = local read "数据14"() -> (w316:dbl[])
                  n185 = local write "输出数组9"(w296) -> ()
                  n186 = local write "输出数组12"(w293) -> ()
                  n187 = local write "输出数组2"(w303) -> ()
                  n188 = local write "输出数组3"(w302) -> ()
                  n189 = local read "数据13"() -> (w318:dbl[])
                  n190 = local read "数据16"() -> (w310:dbl[])
                  n191 = local write "输出数组14"(w291) -> ()
                  n192 = local write "输出数组15"(w290) -> ()
                  n193 = local read "数据10"() -> (w327:dbl[])
                  n194 = local write "输出数组5"(w300) -> ()
                  n195 = local read "数据12"() -> (w321:dbl[])
                  n196 = local write "输出数组1"(w306) -> ()
                  n197 = local write "输出数组10"(w295) -> ()
                  n198 = local write "输出数组11"(w294) -> ()
                  n199 = local read "数据2"() -> (w351:dbl[])
                  n200 = local read "数据7"() -> (w336:dbl[])
                  n201 = local read "数据6"() -> (w339:dbl[])
                  n202 = local read "数据8"() -> (w333:dbl[])
                  n203 = local read "数据5"() -> (w342:dbl[])
                  n204 = local read "数据11"() -> (w324:dbl[])
                  n205 = local read "数据3"() -> (w348:dbl[])
                  n206 = local read "数据4"() -> (w345:dbl[])
                  n207 = local read "数据9"() -> (w330:dbl[])
                  n208 = local read "数据1"() -> (w353:dbl[])
                  n209 = Insert Into Array(array=w316, new element=w315) -> (w314:dbl[])  [unwired: 1 in]
                  n210 = Array Size(array=w291) -> (size(s)=→"AI 13 size(s)":i32)
                  n211 = Array Size(array=w290) -> (size(s)=→"AI 14 size(s)":i32)
                  n212 = Insert Into Array(array=w312, new element=w313) -> (w311:dbl[])  [unwired: 1 in]
                  n213 = Insert Into Array(array=w310, new element=w309) -> (w308:dbl[])  [unwired: 1 in]
                  n214 = Array Size(array=w289) -> (size(s)=→"AI 15 size(s)":i32)
                  n215 = Array Size(array=w292) -> (size(s)=→"AI 12 size(s)":i32)
                  n216 = Insert Into Array(array=w318, new element=w319) -> (w317:dbl[])  [unwired: 1 in]
                  n217 = Insert Into Array(array=w321, new element=w322) -> (w320:dbl[])  [unwired: 1 in]
                  n218 = Array Size(array=w295) -> (size(s)=→"AI 9 size(s)":i32)
                  n219 = Insert Into Array(array=w327, new element=w328) -> (w326:dbl[])  [unwired: 1 in]
                  n220 = Array Size(array=w293) -> (size(s)=→"AI 11 size(s)":i32)
                  n221 = Array Size(array=w294) -> (size(s)=→"AI 10 size(s)":i32)
                  n222 = Insert Into Array(array=w324, new element=w325) -> (w323:dbl[])  [unwired: 1 in]
                  n223 = Array Size(array=w296) -> (size(s)=→"AI 8 size(s)":i32)
                  n224 = Insert Into Array(array=w330, new element=w331) -> (w329:dbl[])  [unwired: 1 in]
                  n225 = Array Size(array=w306) -> (size(s)=→"AI 0 size(s)":i32)
                  n226 = Insert Into Array(array=w353, new element=w354) -> (w305:dbl[])  [unwired: 1 in]
                  "波形图 3" <- w305
                  n227 = Array Size(array=w303) -> (size(s)=→"AI 1 size(s)":i32)
                  n228 = Insert Into Array(array=w351, new element=w352) -> (w350:dbl[])  [unwired: 1 in]
                  n229 = Insert Into Array(array=w348, new element=w349) -> (w347:dbl[])  [unwired: 1 in]
                  n230 = Array Size(array=w302) -> (size(s)=→"AI 2 size(s)":i32)
                  n231 = Insert Into Array(array=w333, new element=w334) -> (w332:dbl[])  [unwired: 1 in]
                  n232 = Array Size(array=w298) -> (size(s)=→"AI 7 size(s)":i32)
                  n233 = Array Size(array=w301) -> (size(s)=→"AI 3 size(s)":i32)
                  n234 = Insert Into Array(array=w345, new element=w346) -> (w344:dbl[])  [unwired: 1 in]
                  n235 = Array Size(array=w300) -> (size(s)=→"AI 4 size(s)":i32)
                  n236 = Insert Into Array(array=w342, new element=w343) -> (w341:dbl[])  [unwired: 1 in]
                  n237 = Insert Into Array(array=w336, new element=w337) -> (w335:dbl[])  [unwired: 1 in]
                  n238 = Array Size(array=w297) -> (size(s)=→"AI 6 size(s)":i32)
                  n239 = Array Size(array=w299) -> (size(s)=→"AI 5 size(s)":i32)
                  n240 = Insert Into Array(array=w339, new element=w340) -> (w338:dbl[])  [unwired: 1 in]
                  n241 = local write "数据14"(w314) -> ()
                  n242 = local write "数据15"(w311) -> ()
                  n243 = local write "数据16"(w308) -> ()
                  n244 = local write "数据13"(w317) -> ()
                  n245 = local write "数据12"(w320) -> ()
                  n246 = local write "数据10"(w326) -> ()
                  n247 = local write "数据11"(w323) -> ()
                  n248 = local write "数据3"(w347) -> ()
                  n249 = local write "数据1"(w305) -> ()
                  n250 = local write "数据9"(w329) -> ()
                  n251 = local write "数据2"(w350) -> ()
                  n252 = local write "数据7"(w335) -> ()
                  n253 = local write "数据8"(w332) -> ()
                  n254 = local write "数据4"(w344) -> ()
                  n255 = local write "数据5"(w341) -> ()
                  n256 = local write "数据6"(w338) -> ()
                  n257 = local write "过程提示"("正在采集数据！！！" ("过程提示")) -> ()
                }
                frame #1 {
                  n258 = local read "AI 0 size(s)"() -> (w413:i32)
                  n259 = local read "采样次数"() -> (w411:u32)
                  n260 = local read "采样率"() -> (w410:u32)
                  n261 = Multiply(x=w411, y=w410) -> (x*y=w409:u32)
                  n262 = Equal?(x=w413, y=w409) -> (x = y?=w412:bool)
                  n263 = case shown="真" w412 {
                    frame False {
                    }
                    frame True {
                      n264 = local read "数据处理及上传控制"() -> (w417:i32)
                      n265 = Increment(x=w417) -> (x+1=w416:i32)
                      n266 = local write "数据处理及上传控制"(w416) -> ()
                    }
                  }
                }
              }
            }
          }
          frame #1 {
            # "数据上传到数据库"
            n267 = local read "数据处理及上传控制"() -> (w421:i32)
            n268 = local read "上传到数据库"() -> (w422:bool)
            n269 = Greater Or Equal?(x=w421, y=2) -> (x >= y?=w419:bool)
            n270 = And(x=w422, y=w419) -> (x .and. y?=w418:bool)
            n271 = case shown="真" w418 {
              tunnel: w424 -> [_ w428]
              tunnel: w423 -> [_ w429]
              frame False {
              }
              frame True {
                n272 = local read "采样次数"() -> (w426:u32)
                n273 = local read "采样率"() -> (w425:u32)
                n274 = Multiply(x=w425, y=w426) -> (x*y=w427:u32)
                n275 = stacked-sequence {
                  tunnel: w429 -> [_ w433 w459 w483 w508 w533 w558 w583 w608 w633 w658 w683 w708 w733 w758 w783 w808]
                  tunnel: w428 -> [_ w434 w458 w484 w509 w534 w559 w584 w609 w634 w659 w684 w709 w734 w759 w784 w809]
                  tunnel: w427 -> [_ w431 w456 w481 w506 w531 w556 w581 w606 w631 w656 w681 w706 w731 w756 w781 w806]
                  frame #0 {
                    n276 = local write "过程提示"("正在将数据保存到数据库中！！！" ("过程提示")) -> ()
                  }
                  frame #1 {
                    n277 = local read "AI0"() -> (w432:bool)
                    n278 = case shown="真" w432 {
                      tunnel: w434 -> [_ w444]
                      tunnel: w433 -> [_ w446]
                      tunnel: w431 -> [_ w435]
                      frame False {
                      }
                      frame True {
                        n279 = local read "输出数组1"() -> (w436:dbl[])
                        n280 = local read "字符串"() -> (w443:string)
                        n281 = for {
                          N: w435 -> [_]
                          tunnel: w436 -> [w452] mode=indexing
                          shift-right: [w450] -> w442
                          shift-left: w443 -> [w449]
                          w451 = T3 0 items=["两端", "字符串首端", "字符串末端"] ("location (both)")
                          n282 = Number To Fractional String(number=w452, width (-)=i16 6 ("宽度(-)")) -> (F-format string=w455:string)  [unwired: 2 in]
                          n283 = call <vilib>:"Trim Whitespace.vi"("string"=w455, "location (both)"=w451) -> ("trimmed string"=w453:string)
                          n284 = Concatenate Strings(w449, "('", w453, "')," ("字符串")) -> (w450:string)
                        }
                        n285 = String Length(string=w442) -> (length=w438:i32)
                        n286 = Decrement(x=w438) -> (x-1=w437:i32)
                        n287 = String Subset(string=w442, length (rest)=w437) -> (substring=w440:string)  [unwired: 1 in]
                        n288 = Concatenate Strings("insert into s1(value) values ", w440) -> (w439:string)
                        n289 = call "SQL Execute.vi"("error in (no error)"=w446, "Return Data (T)"=FALSE, "Command Text"=w439, "ADODB._Connection In"=w444) -> ()  [unwired: 4 in, 4 out]
                      }
                    }
                  }
                  frame #2 {
                    n290 = local read "AI1"() -> (w457:bool)
                    n291 = case shown="真" w457 {
                      tunnel: w459 -> [_ w465]
                      tunnel: w458 -> [_ w466]
                      tunnel: w456 -> [_ w460]
                      frame False {
                      }
                      frame True {
                        n292 = local read "字符串"() -> (w464:string)
                        n293 = local read "输出数组2"() -> (w461:dbl[])
                        n294 = for {
                          N: w460 -> [_]
                          shift-right: [w476] -> w470
                          shift-left: w464 -> [w475]
                          tunnel: w461 -> [w472] mode=indexing
                          w477 = T3 0 items=["两端", "字符串首端", "字符串末端"] ("location (both)")
                          n295 = Number To Fractional String(number=w472, width (-)=i16 6 ("宽度(-)")) -> (F-format string=w480:string)  [unwired: 2 in]
                          n296 = call <vilib>:"Trim Whitespace.vi"("string"=w480, "location (both)"=w477) -> ("trimmed string"=w478:string)
                          n297 = Concatenate Strings(w475, "('", w478, "')," ("字符串")) -> (w476:string)
                        }
                        n298 = String Length(string=w470) -> (length=w463:i32)
                        n299 = Decrement(x=w463) -> (x-1=w462:i32)
                        n300 = String Subset(string=w470, length (rest)=w462) -> (substring=w468:string)  [unwired: 1 in]
                        n301 = Concatenate Strings("insert into s2 (value) values ", w468) -> (w467:string)
                        n302 = call "SQL Execute.vi"("error in (no error)"=w465, "Return Data (T)"=FALSE, "Command Text"=w467, "ADODB._Connection In"=w466) -> ()  [unwired: 4 in, 4 out]
                      }
                    }
                  }
                  frame #3 {
                    n303 = local read "AI2"() -> (w482:bool)
                    n304 = case shown="真" w482 {
                      tunnel: w484 -> [_ w491]
                      tunnel: w483 -> [_ w490]
                      tunnel: w481 -> [_ w485]
                      frame False {
                      }
                      frame True {
                        n305 = local read "输出数组3"() -> (w486:dbl[])
                        n306 = local read "字符串"() -> (w489:string)
                        n307 = for {
                          N: w485 -> [_]
                          shift-right: [w501] -> w495
                          shift-left: w489 -> [w500]
                          tunnel: w486 -> [w497] mode=indexing
                          w502 = T3 0 items=["两端", "字符串首端", "字符串末端"] ("location (both)")
                          n308 = Number To Fractional String(number=w497, width (-)=i16 6 ("宽度(-)")) -> (F-format string=w505:string)  [unwired: 2 in]
                          n309 = call <vilib>:"Trim Whitespace.vi"("string"=w505, "location (both)"=w502) -> ("trimmed string"=w503:string)
                          n310 = Concatenate Strings(w500, "('", w503, "')," ("字符串")) -> (w501:string)
                        }
                        n311 = String Length(string=w495) -> (length=w488:i32)
                        n312 = Decrement(x=w488) -> (x-1=w487:i32)
                        n313 = String Subset(string=w495, length (rest)=w487) -> (substring=w493:string)  [unwired: 1 in]
                        n314 = Concatenate Strings("insert into s3 (value) values ", w493) -> (w492:string)
                        n315 = call "SQL Execute.vi"("error in (no error)"=w490, "Return Data (T)"=FALSE, "Command Text"=w492, "ADODB._Connection In"=w491) -> ()  [unwired: 4 in, 4 out]
                      }
                    }
                  }
                  frame #4 {
                    n316 = local read "AI3"() -> (w507:bool)
                    n317 = case shown="真" w507 {
                      tunnel: w509 -> [_ w516]
                      tunnel: w508 -> [_ w515]
                      tunnel: w506 -> [_ w510]
                      frame False {
                      }
                      frame True {
                        n318 = local read "输出数组4"() -> (w511:dbl[])
                        n319 = local read "字符串"() -> (w514:string)
                        n320 = for {
                          N: w510 -> [_]
                          shift-right: [w526] -> w520
                          shift-left: w514 -> [w525]
                          tunnel: w511 -> [w522] mode=indexing
                          w527 = T3 0 items=["两端", "字符串首端", "字符串末端"] ("location (both)")
                          n321 = Number To Fractional String(number=w522, width (-)=i16 6 ("宽度(-)")) -> (F-format string=w530:string)  [unwired: 2 in]
                          n322 = call <vilib>:"Trim Whitespace.vi"("string"=w530, "location (both)"=w527) -> ("trimmed string"=w528:string)
                          n323 = Concatenate Strings(w525, "('", w528, "')," ("字符串")) -> (w526:string)
                        }
                        n324 = String Length(string=w520) -> (length=w513:i32)
                        n325 = Decrement(x=w513) -> (x-1=w512:i32)
                        n326 = String Subset(string=w520, length (rest)=w512) -> (substring=w518:string)  [unwired: 1 in]
                        n327 = Concatenate Strings("insert into s4(value) values ", w518) -> (w517:string)
                        n328 = call "SQL Execute.vi"("error in (no error)"=w515, "Return Data (T)"=FALSE, "Command Text"=w517, "ADODB._Connection In"=w516) -> ()  [unwired: 4 in, 4 out]
                      }
                    }
                  }
                  frame #5 {
                    n329 = local read "AI4"() -> (w532:bool)
                    n330 = case shown="真" w532 {
                      tunnel: w534 -> [_ w540]
                      tunnel: w533 -> [_ w539]
                      tunnel: w531 -> [_ w535]
                      frame False {
                      }
                      frame True {
                        n331 = local read "输出数组5"() -> (w541:dbl[])
                        n332 = local read "字符串"() -> (w538:string)
                        n333 = for {
                          N: w535 -> [_]
                          shift-right: [w551] -> w545
                          shift-left: w538 -> [w550]
                          tunnel: w541 -> [w547] mode=indexing
                          w552 = T3 0 items=["两端", "字符串首端", "字符串末端"] ("location (both)")
                          n334 = Number To Fractional String(number=w547, width (-)=i16 6 ("宽度(-)")) -> (F-format string=w555:string)  [unwired: 2 in]
                          n335 = call <vilib>:"Trim Whitespace.vi"("string"=w555, "location (both)"=w552) -> ("trimmed string"=w553:string)
                          n336 = Concatenate Strings(w550, "('", w553, "')," ("字符串")) -> (w551:string)
                        }
                        n337 = String Length(string=w545) -> (length=w536:i32)
                        n338 = Decrement(x=w536) -> (x-1=w537:i32)
                        n339 = String Subset(string=w545, length (rest)=w537) -> (substring=w543:string)  [unwired: 1 in]
                        n340 = Concatenate Strings("insert into s5(value) values ", w543) -> (w542:string)
                        n341 = call "SQL Execute.vi"("error in (no error)"=w539, "Return Data (T)"=FALSE, "Command Text"=w542, "ADODB._Connection In"=w540) -> ()  [unwired: 4 in, 4 out]
                      }
                    }
                  }
                  frame #6 {
                    n342 = local read "AI5"() -> (w557:bool)
                    n343 = case shown="真" w557 {
                      tunnel: w559 -> [_ w565]
                      tunnel: w558 -> [_ w564]
                      tunnel: w556 -> [_ w560]
                      frame False {
                      }
                      frame True {
                        n344 = local read "字符串"() -> (w566:string)
                        n345 = local read "输出数组6"() -> (w561:dbl[])
                        n346 = for {
                          N: w560 -> [_]
                          shift-right: [w576] -> w570
                          shift-left: w566 -> [w575]
                          tunnel: w561 -> [w572] mode=indexing
                          w577 = T3 0 items=["两端", "字符串首端", "字符串末端"] ("location (both)")
                          n347 = Number To Fractional String(number=w572, width (-)=i16 6 ("宽度(-)")) -> (F-format string=w580:string)  [unwired: 2 in]
                          n348 = call <vilib>:"Trim Whitespace.vi"("string"=w580, "location (both)"=w577) -> ("trimmed string"=w578:string)
                          n349 = Concatenate Strings(w575, "('", w578, "')," ("字符串")) -> (w576:string)
                        }
                        n350 = String Length(string=w570) -> (length=w562:i32)
                        n351 = Decrement(x=w562) -> (x-1=w563:i32)
                        n352 = String Subset(string=w570, length (rest)=w563) -> (substring=w568:string)  [unwired: 1 in]
                        n353 = Concatenate Strings("insert into s6(value) values ", w568) -> (w567:string)
                        n354 = call "SQL Execute.vi"("error in (no error)"=w564, "Return Data (T)"=FALSE, "Command Text"=w567, "ADODB._Connection In"=w565) -> ()  [unwired: 4 in, 4 out]
                      }
                    }
                  }
                  frame #7 {
                    n355 = local read "AI6"() -> (w582:bool)
                    n356 = case shown="真" w582 {
                      tunnel: w584 -> [_ w590]
                      tunnel: w583 -> [_ w589]
                      tunnel: w581 -> [_ w585]
                      frame False {
                      }
                      frame True {
                        n357 = local read "输出数组7"() -> (w586:dbl[])
                        n358 = local read "字符串"() -> (w591:string)
                        n359 = for {
                          N: w585 -> [_]
                          shift-right: [w601] -> w595
                          shift-left: w591 -> [w600]
                          tunnel: w586 -> [w597] mode=indexing
                          w602 = T3 0 items=["两端", "字符串首端", "字符串末端"] ("location (both)")
                          n360 = Number To Fractional String(number=w597, width (-)=i16 6 ("宽度(-)")) -> (F-format string=w605:string)  [unwired: 2 in]
                          n361 = call <vilib>:"Trim Whitespace.vi"("string"=w605, "location (both)"=w602) -> ("trimmed string"=w603:string)
                          n362 = Concatenate Strings(w600, "('", w603, "')," ("字符串")) -> (w601:string)
                        }
                        n363 = String Length(string=w595) -> (length=w587:i32)
                        n364 = Decrement(x=w587) -> (x-1=w588:i32)
                        n365 = String Subset(string=w595, length (rest)=w588) -> (substring=w593:string)  [unwired: 1 in]
                        n366 = Concatenate Strings("insert into s7(value) values ", w593) -> (w592:string)
                        n367 = call "SQL Execute.vi"("error in (no error)"=w589, "Return Data (T)"=FALSE, "Command Text"=w592, "ADODB._Connection In"=w590) -> ()  [unwired: 4 in, 4 out]
                      }
                    }
                  }
                  frame #8 {
                    n368 = local read "AI7"() -> (w607:bool)
                    n369 = case shown="真" w607 {
                      tunnel: w609 -> [_ w616]
                      tunnel: w608 -> [_ w615]
                      tunnel: w606 -> [_ w610]
                      frame False {
                      }
                      frame True {
                        n370 = local read "输出数组8"() -> (w611:dbl[])
                        n371 = local read "字符串"() -> (w614:string)
                        n372 = for {
                          N: w610 -> [_]
                          shift-right: [w626] -> w620
                          shift-left: w614 -> [w625]
                          tunnel: w611 -> [w622] mode=indexing
                          w627 = T3 0 items=["两端", "字符串首端", "字符串末端"] ("location (both)")
                          n373 = Number To Fractional String(number=w622, width (-)=i16 6 ("宽度(-)")) -> (F-format string=w630:string)  [unwired: 2 in]
                          n374 = call <vilib>:"Trim Whitespace.vi"("string"=w630, "location (both)"=w627) -> ("trimmed string"=w628:string)
                          n375 = Concatenate Strings(w625, "('", w628, "')," ("字符串")) -> (w626:string)
                        }
                        n376 = String Length(string=w620) -> (length=w612:i32)
                        n377 = Decrement(x=w612) -> (x-1=w613:i32)
                        n378 = String Subset(string=w620, length (rest)=w613) -> (substring=w618:string)  [unwired: 1 in]
                        n379 = Concatenate Strings("insert into s8(value) values ", w618) -> (w617:string)
                        n380 = call "SQL Execute.vi"("error in (no error)"=w615, "Return Data (T)"=FALSE, "Command Text"=w617, "ADODB._Connection In"=w616) -> ()  [unwired: 4 in, 4 out]
                      }
                    }
                  }
                  frame #9 {
                    n381 = local read "AI8"() -> (w632:bool)
                    n382 = case shown="真" w632 {
                      tunnel: w634 -> [_ w641]
                      tunnel: w633 -> [_ w640]
                      tunnel: w631 -> [_ w635]
                      frame False {
                      }
                      frame True {
                        n383 = local read "输出数组9"() -> (w636:dbl[])
                        n384 = local read "字符串"() -> (w639:string)
                        n385 = for {
                          N: w635 -> [_]
                          shift-right: [w651] -> w645
                          shift-left: w639 -> [w650]
                          tunnel: w636 -> [w647] mode=indexing
                          w652 = T3 0 items=["两端", "字符串首端", "字符串末端"] ("location (both)")
                          n386 = Number To Fractional String(number=w647, width (-)=i16 6 ("宽度(-)")) -> (F-format string=w655:string)  [unwired: 2 in]
                          n387 = call <vilib>:"Trim Whitespace.vi"("string"=w655, "location (both)"=w652) -> ("trimmed string"=w653:string)
                          n388 = Concatenate Strings(w650, "('", w653, "')," ("字符串")) -> (w651:string)
                        }
                        n389 = String Length(string=w645) -> (length=w637:i32)
                        n390 = Decrement(x=w637) -> (x-1=w638:i32)
                        n391 = String Subset(string=w645, length (rest)=w638) -> (substring=w643:string)  [unwired: 1 in]
                        n392 = Concatenate Strings("insert into s9(value) values ", w643) -> (w642:string)
                        n393 = call "SQL Execute.vi"("error in (no error)"=w640, "Return Data (T)"=FALSE, "Command Text"=w642, "ADODB._Connection In"=w641) -> ()  [unwired: 4 in, 4 out]
                      }
                    }
                  }
                  frame #10 {
                    n394 = local read "AI9"() -> (w657:bool)
                    n395 = case shown="真" w657 {
                      tunnel: w659 -> [_ w665]
                      tunnel: w658 -> [_ w666]
                      tunnel: w656 -> [_ w660]
                      frame False {
                      }
                      frame True {
                        n396 = local read "输出数组10"() -> (w661:dbl[])
                        n397 = local read "字符串"() -> (w664:string)
                        n398 = for {
                          N: w660 -> [_]
                          shift-right: [w676] -> w670
                          shift-left: w664 -> [w675]
                          tunnel: w661 -> [w672] mode=indexing
                          w677 = T3 0 items=["两端", "字符串首端", "字符串末端"] ("location (both)")
                          n399 = Number To Fractional String(number=w672, width (-)=i16 6 ("宽度(-)")) -> (F-format string=w680:string)  [unwired: 2 in]
                          n400 = call <vilib>:"Trim Whitespace.vi"("string"=w680, "location (both)"=w677) -> ("trimmed string"=w678:string)
                          n401 = Concatenate Strings(w675, "('", w678, "')," ("字符串")) -> (w676:string)
                        }
                        n402 = String Length(string=w670) -> (length=w662:i32)
                        n403 = Decrement(x=w662) -> (x-1=w663:i32)
                        n404 = String Subset(string=w670, length (rest)=w663) -> (substring=w668:string)  [unwired: 1 in]
                        n405 = Concatenate Strings("insert into s10(value) values ", w668) -> (w667:string)
                        n406 = call "SQL Execute.vi"("error in (no error)"=w666, "Return Data (T)"=FALSE, "Command Text"=w667, "ADODB._Connection In"=w665) -> ()  [unwired: 4 in, 4 out]
                      }
                    }
                  }
                  frame #11 {
                    n407 = local read "AI10"() -> (w682:bool)
                    n408 = case shown="真" w682 {
                      tunnel: w684 -> [_ w691]
                      tunnel: w683 -> [_ w690]
                      tunnel: w681 -> [_ w685]
                      frame False {
                      }
                      frame True {
                        n409 = local read "输出数组11"() -> (w686:dbl[])
                        n410 = local read "字符串"() -> (w689:string)
                        n411 = for {
                          N: w685 -> [_]
                          shift-right: [w701] -> w695
                          shift-left: w689 -> [w700]
                          tunnel: w686 -> [w697] mode=indexing
                          w702 = T3 0 items=["两端", "字符串首端", "字符串末端"] ("location (both)")
                          n412 = Number To Fractional String(number=w697, width (-)=i16 6 ("宽度(-)")) -> (F-format string=w705:string)  [unwired: 2 in]
                          n413 = call <vilib>:"Trim Whitespace.vi"("string"=w705, "location (both)"=w702) -> ("trimmed string"=w703:string)
                          n414 = Concatenate Strings(w700, "('", w703, "')," ("字符串")) -> (w701:string)
                        }
                        n415 = String Length(string=w695) -> (length=w687:i32)
                        n416 = Decrement(x=w687) -> (x-1=w688:i32)
                        n417 = String Subset(string=w695, length (rest)=w688) -> (substring=w693:string)  [unwired: 1 in]
                        n418 = Concatenate Strings("insert into s11(value) values ", w693) -> (w692:string)
                        n419 = call "SQL Execute.vi"("error in (no error)"=w690, "Return Data (T)"=FALSE, "Command Text"=w692, "ADODB._Connection In"=w691) -> ()  [unwired: 4 in, 4 out]
                      }
                    }
                  }
                  frame #12 {
                    n420 = local read "AI11"() -> (w707:bool)
                    n421 = case shown="真" w707 {
                      tunnel: w709 -> [_ w715]
                      tunnel: w708 -> [_ w714]
                      tunnel: w706 -> [_ w710]
                      frame False {
                      }
                      frame True {
                        n422 = local read "输出数组12"() -> (w711:dbl[])
                        n423 = local read "字符串"() -> (w716:string)
                        n424 = for {
                          N: w710 -> [_]
                          shift-right: [w726] -> w720
                          shift-left: w716 -> [w725]
                          tunnel: w711 -> [w722] mode=indexing
                          w727 = T3 0 items=["两端", "字符串首端", "字符串末端"] ("location (both)")
                          n425 = Number To Fractional String(number=w722, width (-)=i16 6 ("宽度(-)")) -> (F-format string=w730:string)  [unwired: 2 in]
                          n426 = call <vilib>:"Trim Whitespace.vi"("string"=w730, "location (both)"=w727) -> ("trimmed string"=w728:string)
                          n427 = Concatenate Strings(w725, "('", w728, "')," ("字符串")) -> (w726:string)
                        }
                        n428 = String Length(string=w720) -> (length=w712:i32)
                        n429 = Decrement(x=w712) -> (x-1=w713:i32)
                        n430 = String Subset(string=w720, length (rest)=w713) -> (substring=w718:string)  [unwired: 1 in]
                        n431 = Concatenate Strings("insert into s12(value) values ", w718) -> (w717:string)
                        n432 = call "SQL Execute.vi"("error in (no error)"=w714, "Return Data (T)"=FALSE, "Command Text"=w717, "ADODB._Connection In"=w715) -> ()  [unwired: 4 in, 4 out]
                      }
                    }
                  }
                  frame #13 {
                    n433 = local read "AI12"() -> (w732:bool)
                    n434 = case shown="真" w732 {
                      tunnel: w734 -> [_ w740]
                      tunnel: w733 -> [_ w739]
                      tunnel: w731 -> [_ w735]
                      frame False {
                      }
                      frame True {
                        n435 = local read "输出数组13"() -> (w736:dbl[])
                        n436 = local read "字符串"() -> (w741:string)
                        n437 = for {
                          N: w735 -> [_]
                          shift-right: [w751] -> w745
                          shift-left: w741 -> [w750]
                          tunnel: w736 -> [w747] mode=indexing
                          w752 = T3 0 items=["两端", "字符串首端", "字符串末端"] ("location (both)")
                          n438 = Number To Fractional String(number=w747, width (-)=i16 6 ("宽度(-)")) -> (F-format string=w755:string)  [unwired: 2 in]
                          n439 = call <vilib>:"Trim Whitespace.vi"("string"=w755, "location (both)"=w752) -> ("trimmed string"=w753:string)
                          n440 = Concatenate Strings(w750, "('", w753, "')," ("字符串")) -> (w751:string)
                        }
                        n441 = String Length(string=w745) -> (length=w737:i32)
                        n442 = Decrement(x=w737) -> (x-1=w738:i32)
                        n443 = String Subset(string=w745, length (rest)=w738) -> (substring=w743:string)  [unwired: 1 in]
                        n444 = Concatenate Strings("insert into s13(value) values ", w743) -> (w742:string)
                        n445 = call "SQL Execute.vi"("error in (no error)"=w739, "Return Data (T)"=FALSE, "Command Text"=w742, "ADODB._Connection In"=w740) -> ()  [unwired: 4 in, 4 out]
                      }
                    }
                  }
                  frame #14 {
                    n446 = local read "AI13"() -> (w757:bool)
                    n447 = case shown="真" w757 {
                      tunnel: w759 -> [_ w766]
                      tunnel: w758 -> [_ w765]
                      tunnel: w756 -> [_ w760]
                      frame False {
                      }
                      frame True {
                        n448 = local read "输出数组14"() -> (w761:dbl[])
                        n449 = local read "字符串"() -> (w764:string)
                        n450 = for {
                          N: w760 -> [_]
                          shift-right: [w776] -> w770
                          shift-left: w764 -> [w775]
                          tunnel: w761 -> [w772] mode=indexing
                          w777 = T3 0 items=["两端", "字符串首端", "字符串末端"] ("location (both)")
                          n451 = Number To Fractional String(number=w772, width (-)=i16 6 ("宽度(-)")) -> (F-format string=w780:string)  [unwired: 2 in]
                          n452 = call <vilib>:"Trim Whitespace.vi"("string"=w780, "location (both)"=w777) -> ("trimmed string"=w778:string)
                          n453 = Concatenate Strings(w775, "('", w778, "')," ("字符串")) -> (w776:string)
                        }
                        n454 = String Length(string=w770) -> (length=w762:i32)
                        n455 = Decrement(x=w762) -> (x-1=w763:i32)
                        n456 = String Subset(string=w770, length (rest)=w763) -> (substring=w768:string)  [unwired: 1 in]
                        n457 = Concatenate Strings("insert into s14(value) values ", w768) -> (w767:string)
                        n458 = call "SQL Execute.vi"("error in (no error)"=w765, "Return Data (T)"=FALSE, "Command Text"=w767, "ADODB._Connection In"=w766) -> ()  [unwired: 4 in, 4 out]
                      }
                    }
                  }
                  frame #15 {
                    n459 = local read "AI14"() -> (w782:bool)
                    n460 = case shown="真" w782 {
                      tunnel: w784 -> [_ w790]
                      tunnel: w783 -> [_ w789]
                      tunnel: w781 -> [_ w785]
                      frame False {
                      }
                      frame True {
                        n461 = local read "输出数组15"() -> (w786:dbl[])
                        n462 = local read "字符串"() -> (w791:string)
                        n463 = for {
                          N: w785 -> [_]
                          shift-right: [w801] -> w795
                          shift-left: w791 -> [w800]
                          tunnel: w786 -> [w797] mode=indexing
                          w802 = T3 0 items=["两端", "字符串首端", "字符串末端"] ("location (both)")
                          n464 = Number To Fractional String(number=w797, width (-)=i16 6 ("宽度(-)")) -> (F-format string=w805:string)  [unwired: 2 in]
                          n465 = call <vilib>:"Trim Whitespace.vi"("string"=w805, "location (both)"=w802) -> ("trimmed string"=w803:string)
                          n466 = Concatenate Strings(w800, "('", w803, "')," ("字符串")) -> (w801:string)
                        }
                        n467 = String Length(string=w795) -> (length=w787:i32)
                        n468 = Decrement(x=w787) -> (x-1=w788:i32)
                        n469 = String Subset(string=w795, length (rest)=w788) -> (substring=w793:string)  [unwired: 1 in]
                        n470 = Concatenate Strings("insert into s15(value) values ", w793) -> (w792:string)
                        n471 = call "SQL Execute.vi"("error in (no error)"=w789, "Return Data (T)"=FALSE, "Command Text"=w792, "ADODB._Connection In"=w790) -> ()  [unwired: 4 in, 4 out]
                      }
                    }
                  }
                  frame #16 {
                    n472 = local read "AI15"() -> (w807:bool)
                    n473 = case shown="真" w807 {
                      tunnel: w809 -> [_ w816]
                      tunnel: w808 -> [_ w815]
                      tunnel: w806 -> [_ w810]
                      frame False {
                      }
                      frame True {
                        n474 = local read "输出数组16"() -> (w812:dbl[])
                        n475 = local read "字符串"() -> (w811:string)
                        n476 = for {
                          N: w810 -> [_]
                          shift-right: [w826] -> w820
                          shift-left: w811 -> [w825]
                          tunnel: w812 -> [w822] mode=indexing
                          w827 = T3 0 items=["两端", "字符串首端", "字符串末端"] ("location (both)")
                          n477 = Number To Fractional String(number=w822, width (-)=i16 6 ("宽度(-)")) -> (F-format string=w830:string)  [unwired: 2 in]
                          n478 = call <vilib>:"Trim Whitespace.vi"("string"=w830, "location (both)"=w827) -> ("trimmed string"=w828:string)
                          n479 = Concatenate Strings(w825, "('", w828, "')," ("字符串")) -> (w826:string)
                        }
                        n480 = String Length(string=w820) -> (length=w814:i32)
                        n481 = Decrement(x=w814) -> (x-1=w813:i32)
                        n482 = String Subset(string=w820, length (rest)=w813) -> (substring=w818:string)  [unwired: 1 in]
                        n483 = Concatenate Strings("insert into s1(value) values ", w818) -> (w817:string)
                        n484 = call "SQL Execute.vi"("error in (no error)"=w815, "Return Data (T)"=FALSE, "Command Text"=w817, "ADODB._Connection In"=w816) -> ()  [unwired: 4 in, 4 out]
                      }
                    }
                  }
                }
              }
            }
          }
          frame #2 {
            # "数据处理"
            n485 = local read "数据处理及上传控制"() -> (w834:i32)
            n486 = local read "数据处理 2"() -> (w833:bool)
            n487 = Greater Or Equal?(x=w834, y=2) -> (x >= y?=w832:bool)
            n488 = And(x=w833, y=w832) -> (x .and. y?=w831:bool)
            n489 = case shown="真" w831 {
              tunnel: w837 -> [_ w841]
              tunnel: w836 -> [_ w840]
              frame False {
              }
              frame True {
                n490 = local read "sym"() -> (w838:string)
                n491 = local read "lev"() -> (w839:i32)
                n492 = stacked-sequence {
                  tunnel: w841 -> [_ w847 w871 w895 w919 w943 w967 w991 w1015 w1039 w1063 w1087 w1111 w1135 w1159 w1183 w1207]
                  tunnel: w840 -> [_ w846 w870 w894 w918 w942 w966 w990 w1014 w1038 w1062 w1086 w1110 w1134 w1158 w1182 w1206]
                  tunnel: w839 -> [_ w845 w869 w893 w917 w941 w965 w988 w1013 w1037 w1061 w1085 w1108 w1133 w1157 w1181 w1205]
                  tunnel: w838 -> [_ w844 w868 w892 w916 w940 w964 w989 w1012 w1036 w1060 w1084 w1109 w1132 w1156 w1180 w1204]
                  frame #0 {
                    n493 = local write "过程提示"("正在进行数据处理！！！" ("过程提示")) -> ()
                    "布尔" <- TRUE ("布尔")
                  }
                  frame #1 {
                    n494 = local read "AI0"() -> (w848:bool)
                    n495 = case shown="真" w848 {
                      tunnel: w847 -> [_ w852]
                      tunnel: w846 -> [_ w851]
                      tunnel: w845 -> [_ w850]
                      tunnel: w844 -> [_ w849]
                      frame False {
                      }
                      frame True {
                        n496 = flat-sequence {
                          tunnel: w850 -> [w854]
                          tunnel: w849 -> [w853]
                          tunnel: w852 -> [w862]
                          tunnel: w851 -> [w861]
                          frame #0 {
                            n497 = local read "输出数组1"() -> (w859:dbl[])
                            n498 = call "数据处理2.vi"("原始数据文件名"="AI0.csv" ("name or relative path"), "去噪信号保存的文件名"="AI100.csv" ("name or relative path"), "sym"=w853, "数组中的数据（输入）"=w859, "lev"=w854) -> ("字符串（输出）"=→"特征值1":string, "特征值（输出）"=→"AI0特征值" →"AI0特征值 2":dbl[][], "去噪后波形图"=→"AI0去噪后波形图" →"去噪后波形图":dbl[][])  [unwired: 4 in]
                          }
                          frame #1 {
                            n499 = local read "特征值1"() -> (w863:string)
                            n500 = Concatenate Strings("insert into sensor1(value1,value2,value3,value4,value5,value6,value7,value8) values(" ("Command Text"), w863, ");") -> (w865:string)
                            n501 = call "SQL Execute.vi"("error in (no error)"=w861, "Return Data (T)"=FALSE, "Command Text"=w865, "ADODB._Connection In"=w862) -> ()  [unwired: 4 in, 4 out]
                          }
                        }
                      }
                    }
                  }
                  frame #2 {
                    n502 = local read "AI1"() -> (w872:bool)
                    n503 = case shown="真" w872 {
                      tunnel: w871 -> [_ w876]
                      tunnel: w870 -> [_ w875]
                      tunnel: w869 -> [_ w874]
                      tunnel: w868 -> [_ w873]
                      frame False {
                      }
                      frame True {
                        n504 = flat-sequence {
                          tunnel: w874 -> [w878]
                          tunnel: w873 -> [w877]
                          tunnel: w876 -> [w886]
                          tunnel: w875 -> [w885]
                          frame #0 {
                            n505 = local read "输出数组2"() -> (w881:dbl[])
                            n506 = call "数据处理2.vi"("原始数据文件名"="AI1.csv" ("name or relative path"), "去噪信号保存的文件名"="AI101.csv" ("name or relative path"), "sym"=w877, "数组中的数据（输入）"=w881, "lev"=w878) -> ("字符串（输出）"=→"特征值2":string, "特征值（输出）"=→"AI1特征值":dbl[][], "去噪后波形图"=→"AI1去噪后波形图":dbl[][])  [unwired: 4 in]
                          }
                          frame #1 {
                            n507 = local read "特征值2"() -> (w887:string)
                            n508 = Concatenate Strings("insert into sensor2(value1,value2,value3,value4,value5,value6,value7,value8) values(" ("Command Text"), w887, ");") -> (w888:string)
                            n509 = call "SQL Execute.vi"("error in (no error)"=w885, "Return Data (T)"=FALSE, "Command Text"=w888, "ADODB._Connection In"=w886) -> ()  [unwired: 4 in, 4 out]
                          }
                        }
                      }
                    }
                  }
                  frame #3 {
                    n510 = local read "AI2"() -> (w896:bool)
                    n511 = case shown="真" w896 {
                      tunnel: w895 -> [_ w900]
                      tunnel: w894 -> [_ w899]
                      tunnel: w893 -> [_ w898]
                      tunnel: w892 -> [_ w897]
                      frame False {
                      }
                      frame True {
                        n512 = flat-sequence {
                          tunnel: w898 -> [w902]
                          tunnel: w897 -> [w901]
                          tunnel: w900 -> [w910]
                          tunnel: w899 -> [w909]
                          frame #0 {
                            n513 = local read "输出数组3"() -> (w908:dbl[])
                            n514 = call "数据处理2.vi"("原始数据文件名"="AI2.csv" ("name or relative path"), "去噪信号保存的文件名"="AI102.csv" ("name or relative path"), "sym"=w901, "数组中的数据（输入）"=w908, "lev"=w902) -> ("字符串（输出）"=→"特征值3":string, "特征值（输出）"=→"AI2特征值":dbl[][], "去噪后波形图"=→"AI2去噪后波形图":dbl[][])  [unwired: 4 in]
                          }
                          frame #1 {
                            n515 = local read "特征值3"() -> (w911:string)
                            n516 = Concatenate Strings("insert into sensor3(value1,value2,value3,value4,value5,value6,value7,value8) values(" ("Command Text"), w911, ");") -> (w912:string)
                            n517 = call "SQL Execute.vi"("error in (no error)"=w909, "Return Data (T)"=FALSE, "Command Text"=w912, "ADODB._Connection In"=w910) -> ()  [unwired: 4 in, 4 out]
                          }
                        }
                      }
                    }
                  }
                  frame #4 {
                    n518 = local read "AI3"() -> (w920:bool)
                    n519 = case shown="真" w920 {
                      tunnel: w919 -> [_ w924]
                      tunnel: w918 -> [_ w923]
                      tunnel: w917 -> [_ w922]
                      tunnel: w916 -> [_ w921]
                      frame False {
                      }
                      frame True {
                        n520 = flat-sequence {
                          tunnel: w922 -> [w926]
                          tunnel: w921 -> [w925]
                          tunnel: w924 -> [w934]
                          tunnel: w923 -> [w933]
                          frame #0 {
                            n521 = local read "输出数组4"() -> (w929:dbl[])
                            n522 = call "数据处理2.vi"("原始数据文件名"="AI3.csv" ("name or relative path"), "去噪信号保存的文件名"="AI103.csv" ("name or relative path"), "sym"=w925, "数组中的数据（输入）"=w929, "lev"=w926) -> ("字符串（输出）"=→"特征值4":string, "特征值（输出）"=→"AI3特征值":dbl[][], "去噪后波形图"=→"AI3去噪后波形图":dbl[][])  [unwired: 4 in]
                          }
                          frame #1 {
                            n523 = local read "特征值4"() -> (w935:string)
                            n524 = Concatenate Strings("insert into sensor4(value1,value2,value3,value4,value5,value6,value7,value8) values(" ("Command Text"), w935, ");") -> (w936:string)
                            n525 = call "SQL Execute.vi"("error in (no error)"=w933, "Return Data (T)"=FALSE, "Command Text"=w936, "ADODB._Connection In"=w934) -> ()  [unwired: 4 in, 4 out]
                          }
                        }
                      }
                    }
                  }
                  frame #5 {
                    n526 = local read "AI4"() -> (w944:bool)
                    n527 = case shown="真" w944 {
                      tunnel: w943 -> [_ w948]
                      tunnel: w942 -> [_ w947]
                      tunnel: w941 -> [_ w946]
                      tunnel: w940 -> [_ w945]
                      frame False {
                      }
                      frame True {
                        n528 = flat-sequence {
                          tunnel: w946 -> [w950]
                          tunnel: w945 -> [w949]
                          tunnel: w948 -> [w958]
                          tunnel: w947 -> [w957]
                          frame #0 {
                            n529 = local read "输出数组5"() -> (w953:dbl[])
                            n530 = call "数据处理2.vi"("原始数据文件名"="AI4.csv" ("name or relative path"), "去噪信号保存的文件名"="AI104.csv" ("name or relative path"), "sym"=w949, "数组中的数据（输入）"=w953, "lev"=w950) -> ("字符串（输出）"=→"特征值5":string, "特征值（输出）"=→"AI4特征值":dbl[][], "去噪后波形图"=→"AI4去噪后波形图":dbl[][])  [unwired: 4 in]
                          }
                          frame #1 {
                            n531 = local read "特征值5"() -> (w959:string)
                            n532 = Concatenate Strings("insert into sensor5(value1,value2,value3,value4,value5,value6,value7,value8) values(" ("Command Text"), w959, ");") -> (w960:string)
                            n533 = call "SQL Execute.vi"("error in (no error)"=w957, "Return Data (T)"=FALSE, "Command Text"=w960, "ADODB._Connection In"=w958) -> ()  [unwired: 4 in, 4 out]
                          }
                        }
                      }
                    }
                  }
                  frame #6 {
                    n534 = local read "AI5"() -> (w968:bool)
                    n535 = case shown="真" w968 {
                      tunnel: w967 -> [_ w972]
                      tunnel: w966 -> [_ w971]
                      tunnel: w965 -> [_ w970]
                      tunnel: w964 -> [_ w969]
                      frame False {
                      }
                      frame True {
                        n536 = flat-sequence {
                          tunnel: w970 -> [w974]
                          tunnel: w969 -> [w973]
                          tunnel: w972 -> [w982]
                          tunnel: w971 -> [w981]
                          frame #0 {
                            n537 = local read "输出数组6"() -> (w977:dbl[])
                            n538 = call "数据处理2.vi"("原始数据文件名"="AI5.csv" ("name or relative path"), "去噪信号保存的文件名"="AI105.csv" ("name or relative path"), "sym"=w973, "数组中的数据（输入）"=w977, "lev"=w974) -> ("字符串（输出）"=→"特征值6":string, "特征值（输出）"=→"AI5特征值":dbl[][], "去噪后波形图"=→"AI5去噪后波形图":dbl[][])  [unwired: 4 in]
                          }
                          frame #1 {
                            n539 = local read "特征值6"() -> (w983:string)
                            n540 = Concatenate Strings("insert into sensor6(value1,value2,value3,value4,value5,value6,value7,value8) values(" ("Command Text"), w983, ");") -> (w984:string)
                            n541 = call "SQL Execute.vi"("error in (no error)"=w981, "Return Data (T)"=FALSE, "Command Text"=w984, "ADODB._Connection In"=w982) -> ()  [unwired: 4 in, 4 out]
                          }
                        }
                      }
                    }
                  }
                  frame #7 {
                    n542 = local read "AI6"() -> (w992:bool)
                    n543 = case shown="真" w992 {
                      tunnel: w991 -> [_ w996]
                      tunnel: w990 -> [_ w995]
                      tunnel: w989 -> [_ w994]
                      tunnel: w988 -> [_ w993]
                      frame False {
                      }
                      frame True {
                        n544 = flat-sequence {
                          tunnel: w994 -> [w998]
                          tunnel: w993 -> [w997]
                          tunnel: w996 -> [w1006]
                          tunnel: w995 -> [w1005]
                          frame #0 {
                            n545 = local read "输出数组7"() -> (w1001:dbl[])
                            n546 = call "数据处理2.vi"("原始数据文件名"="AI6.csv" ("name or relative path"), "去噪信号保存的文件名"="AI106.csv" ("name or relative path"), "sym"=w998, "数组中的数据（输入）"=w1001, "lev"=w997) -> ("字符串（输出）"=→"特征值7":string, "特征值（输出）"=→"AI6特征值":dbl[][], "去噪后波形图"=→"AI6去噪后波形图":dbl[][])  [unwired: 4 in]
                          }
                          frame #1 {
                            n547 = local read "特征值7"() -> (w1007:string)
                            n548 = Concatenate Strings("insert into sensor7(value1,value2,value3,value4,value5,value6,value7,value8) values(" ("Command Text"), w1007, ");") -> (w1008:string)
                            n549 = call "SQL Execute.vi"("error in (no error)"=w1005, "Return Data (T)"=FALSE, "Command Text"=w1008, "ADODB._Connection In"=w1006) -> ()  [unwired: 4 in, 4 out]
                          }
                        }
                      }
                    }
                  }
                  frame #8 {
                    n550 = local read "AI7"() -> (w1016:bool)
                    n551 = case shown="真" w1016 {
                      tunnel: w1015 -> [_ w1020]
                      tunnel: w1014 -> [_ w1019]
                      tunnel: w1013 -> [_ w1018]
                      tunnel: w1012 -> [_ w1017]
                      frame False {
                      }
                      frame True {
                        n552 = flat-sequence {
                          tunnel: w1018 -> [w1022]
                          tunnel: w1017 -> [w1021]
                          tunnel: w1020 -> [w1030]
                          tunnel: w1019 -> [w1029]
                          frame #0 {
                            n553 = local read "输出数组8"() -> (w1025:dbl[])
                            n554 = call "数据处理2.vi"("原始数据文件名"="AI7.csv" ("name or relative path"), "去噪信号保存的文件名"="AI107.csv" ("name or relative path"), "sym"=w1021, "数组中的数据（输入）"=w1025, "lev"=w1022) -> ("字符串（输出）"=→"特征值8":string, "特征值（输出）"=→"AI7特征值":dbl[][], "去噪后波形图"=→"AI7去噪后波形图":dbl[][])  [unwired: 4 in]
                          }
                          frame #1 {
                            n555 = local read "特征值8"() -> (w1031:string)
                            n556 = Concatenate Strings("insert into sensor8(value1,value2,value3,value4,value5,value6,value7,value8) values(" ("Command Text"), w1031, ");") -> (w1032:string)
                            n557 = call "SQL Execute.vi"("error in (no error)"=w1029, "Return Data (T)"=FALSE, "Command Text"=w1032, "ADODB._Connection In"=w1030) -> ()  [unwired: 4 in, 4 out]
                          }
                        }
                      }
                    }
                  }
                  frame #9 {
                    n558 = local read "AI8"() -> (w1040:bool)
                    n559 = case shown="真" w1040 {
                      tunnel: w1039 -> [_ w1044]
                      tunnel: w1038 -> [_ w1043]
                      tunnel: w1037 -> [_ w1042]
                      tunnel: w1036 -> [_ w1041]
                      frame False {
                      }
                      frame True {
                        n560 = flat-sequence {
                          tunnel: w1042 -> [w1046]
                          tunnel: w1041 -> [w1045]
                          tunnel: w1044 -> [w1054]
                          tunnel: w1043 -> [w1053]
                          frame #0 {
                            n561 = local read "输出数组9"() -> (w1052:dbl[])
                            n562 = call "数据处理2.vi"("原始数据文件名"="AI8.csv" ("name or relative path"), "去噪信号保存的文件名"="AI108.csv" ("name or relative path"), "sym"=w1045, "数组中的数据（输入）"=w1052, "lev"=w1046) -> ("字符串（输出）"=→"特征值9":string, "特征值（输出）"=→"AI8特征值":dbl[][], "去噪后波形图"=→"AI8去噪后波形图":dbl[][])  [unwired: 4 in]
                          }
                          frame #1 {
                            n563 = local read "特征值9"() -> (w1055:string)
                            n564 = Concatenate Strings("insert into sensor9(value1,value2,value3,value4,value5,value6,value7,value8) values(" ("Command Text"), w1055, ");") -> (w1056:string)
                            n565 = call "SQL Execute.vi"("error in (no error)"=w1053, "Return Data (T)"=FALSE, "Command Text"=w1056, "ADODB._Connection In"=w1054) -> ()  [unwired: 4 in, 4 out]
                          }
                        }
                      }
                    }
                  }
                  frame #10 {
                    n566 = local read "AI9"() -> (w1064:bool)
                    n567 = case shown="真" w1064 {
                      tunnel: w1063 -> [_ w1068]
                      tunnel: w1062 -> [_ w1067]
                      tunnel: w1061 -> [_ w1066]
                      tunnel: w1060 -> [_ w1065]
                      frame False {
                      }
                      frame True {
                        n568 = flat-sequence {
                          tunnel: w1066 -> [w1070]
                          tunnel: w1065 -> [w1069]
                          tunnel: w1068 -> [w1078]
                          tunnel: w1067 -> [w1077]
                          frame #0 {
                            n569 = local read "输出数组10"() -> (w1076:dbl[])
                            n570 = call "数据处理2.vi"("原始数据文件名"="AI9.csv" ("name or relative path"), "去噪信号保存的文件名"="AI19.csv" ("name or relative path"), "sym"=w1069, "数组中的数据（输入）"=w1076, "lev"=w1070) -> ("字符串（输出）"=→"特征值10":string, "特征值（输出）"=→"AI9特征值":dbl[][], "去噪后波形图"=→"AI9去噪后波形图":dbl[][])  [unwired: 4 in]
                          }
                          frame #1 {
                            n571 = local read "特征值10"() -> (w1079:string)
                            n572 = Concatenate Strings("insert into sensor10(value1,value2,value3,value4,value5,value6,value7,value8) values(" ("Command Text"), w1079, ");") -> (w1080:string)
                            n573 = call "SQL Execute.vi"("error in (no error)"=w1077, "Return Data (T)"=FALSE, "Command Text"=w1080, "ADODB._Connection In"=w1078) -> ()  [unwired: 4 in, 4 out]
                          }
                        }
                      }
                    }
                  }
                  frame #11 {
                    n574 = local read "AI10"() -> (w1088:bool)
                    n575 = case shown="真" w1088 {
                      tunnel: w1087 -> [_ w1092]
                      tunnel: w1086 -> [_ w1091]
                      tunnel: w1085 -> [_ w1090]
                      tunnel: w1084 -> [_ w1089]
                      frame False {
                      }
                      frame True {
                        n576 = flat-sequence {
                          tunnel: w1090 -> [w1094]
                          tunnel: w1089 -> [w1093]
                          tunnel: w1092 -> [w1102]
                          tunnel: w1091 -> [w1101]
                          frame #0 {
                            n577 = local read "输出数组11"() -> (w1098:dbl[])
                            n578 = call "数据处理2.vi"("原始数据文件名"="AI10.csv" ("name or relative path"), "去噪信号保存的文件名"="AI110.csv" ("name or relative path"), "sym"=w1093, "数组中的数据（输入）"=w1098, "lev"=w1094) -> ("字符串（输出）"=→"特征值11":string, "特征值（输出）"=→"AI10特征值":dbl[][], "去噪后波形图"=→"AI10去噪后波形图":dbl[][])  [unwired: 4 in]
                          }
                          frame #1 {
                            n579 = local read "特征值11"() -> (w1103:string)
                            n580 = Concatenate Strings("insert into sensor11(value1,value2,value3,value4,value5,value6,value7,value8) values(" ("Command Text"), w1103, ");") -> (w1104:string)
                            n581 = call "SQL Execute.vi"("error in (no error)"=w1101, "Return Data (T)"=FALSE, "Command Text"=w1104, "ADODB._Connection In"=w1102) -> ()  [unwired: 4 in, 4 out]
                          }
                        }
                      }
                    }
                  }
                  frame #12 {
                    n582 = local read "AI11"() -> (w1112:bool)
                    n583 = case shown="真" w1112 {
                      tunnel: w1111 -> [_ w1116]
                      tunnel: w1110 -> [_ w1115]
                      tunnel: w1109 -> [_ w1114]
                      tunnel: w1108 -> [_ w1113]
                      frame False {
                      }
                      frame True {
                        n584 = flat-sequence {
                          tunnel: w1114 -> [w1118]
                          tunnel: w1113 -> [w1117]
                          tunnel: w1116 -> [w1126]
                          tunnel: w1115 -> [w1125]
                          frame #0 {
                            n585 = local read "输出数组12"() -> (w1122:dbl[])
                            n586 = call "数据处理2.vi"("原始数据文件名"="AI11.csv" ("name or relative path"), "去噪信号保存的文件名"="AI111.csv" ("name or relative path"), "sym"=w1118, "数组中的数据（输入）"=w1122, "lev"=w1117) -> ("字符串（输出）"=→"特征值12":string, "特征值（输出）"=→"AI11特征值":dbl[][], "去噪后波形图"=→"AI11去噪后波形图":dbl[][])  [unwired: 4 in]
                          }
                          frame #1 {
                            n587 = local read "特征值12"() -> (w1127:string)
                            n588 = Concatenate Strings("insert into sensor12(value1,value2,value3,value4,value5,value6,value7,value8) values(" ("Command Text"), w1127, ");") -> (w1128:string)
                            n589 = call "SQL Execute.vi"("error in (no error)"=w1125, "Return Data (T)"=FALSE, "Command Text"=w1128, "ADODB._Connection In"=w1126) -> ()  [unwired: 4 in, 4 out]
                          }
                        }
                      }
                    }
                  }
                  frame #13 {
                    n590 = local read "AI12"() -> (w1136:bool)
                    n591 = case shown="真" w1136 {
                      tunnel: w1135 -> [_ w1140]
                      tunnel: w1134 -> [_ w1139]
                      tunnel: w1133 -> [_ w1138]
                      tunnel: w1132 -> [_ w1137]
                      frame False {
                      }
                      frame True {
                        n592 = flat-sequence {
                          tunnel: w1138 -> [w1142]
                          tunnel: w1137 -> [w1141]
                          tunnel: w1140 -> [w1150]
                          tunnel: w1139 -> [w1149]
                          frame #0 {
                            n593 = local read "输出数组13"() -> (w1146:dbl[])
                            n594 = call "数据处理2.vi"("原始数据文件名"="AI12.csv" ("name or relative path"), "去噪信号保存的文件名"="AI112.csv" ("name or relative path"), "sym"=w1141, "数组中的数据（输入）"=w1146, "lev"=w1142) -> ("字符串（输出）"=→"特征值13":string, "特征值（输出）"=→"AI12特征值":dbl[][], "去噪后波形图"=→"AI2去噪后波形图":dbl[][])  [unwired: 4 in]
                          }
                          frame #1 {
                            n595 = local read "特征值13"() -> (w1151:string)
                            n596 = Concatenate Strings("insert into sensor13(value1,value2,value3,value4,value5,value6,value7,value8) values(" ("Command Text"), w1151, ");") -> (w1152:string)
                            n597 = call "SQL Execute.vi"("error in (no error)"=w1149, "Return Data (T)"=FALSE, "Command Text"=w1152, "ADODB._Connection In"=w1150) -> ()  [unwired: 4 in, 4 out]
                          }
                        }
                      }
                    }
                  }
                  frame #14 {
                    n598 = local read "AI13"() -> (w1160:bool)
                    n599 = case shown="真" w1160 {
                      tunnel: w1159 -> [_ w1164]
                      tunnel: w1158 -> [_ w1163]
                      tunnel: w1157 -> [_ w1162]
                      tunnel: w1156 -> [_ w1161]
                      frame False {
                      }
                      frame True {
                        n600 = flat-sequence {
                          tunnel: w1162 -> [w1166]
                          tunnel: w1161 -> [w1165]
                          tunnel: w1164 -> [w1174]
                          tunnel: w1163 -> [w1173]
                          frame #0 {
                            n601 = local read "输出数组14"() -> (w1170:dbl[])
                            n602 = call "数据处理2.vi"("原始数据文件名"="AI13.csv" ("name or relative path"), "去噪信号保存的文件名"="AI113.csv" ("name or relative path"), "sym"=w1165, "数组中的数据（输入）"=w1170, "lev"=w1166) -> ("字符串（输出）"=→"特征值14":string, "特征值（输出）"=→"AI13特征值":dbl[][], "去噪后波形图"=→"AI13去噪后波形图":dbl[][])  [unwired: 4 in]
                          }
                          frame #1 {
                            n603 = local read "特征值14"() -> (w1175:string)
                            n604 = Concatenate Strings("insert into sensor14(value1,value2,value3,value4,value5,value6,value7,value8) values(" ("Command Text"), w1175, ");") -> (w1176:string)
                            n605 = call "SQL Execute.vi"("error in (no error)"=w1173, "Return Data (T)"=FALSE, "Command Text"=w1176, "ADODB._Connection In"=w1174) -> ()  [unwired: 4 in, 4 out]
                          }
                        }
                      }
                    }
                  }
                  frame #15 {
                    n606 = local read "AI14"() -> (w1184:bool)
                    n607 = case shown="真" w1184 {
                      tunnel: w1183 -> [_ w1188]
                      tunnel: w1182 -> [_ w1187]
                      tunnel: w1181 -> [_ w1186]
                      tunnel: w1180 -> [_ w1185]
                      frame False {
                      }
                      frame True {
                        n608 = flat-sequence {
                          tunnel: w1186 -> [w1190]
                          tunnel: w1185 -> [w1189]
                          tunnel: w1188 -> [w1198]
                          tunnel: w1187 -> [w1197]
                          frame #0 {
                            n609 = local read "输出数组15"() -> (w1194:dbl[])
                            n610 = call "数据处理2.vi"("原始数据文件名"="AI14.csv" ("name or relative path"), "去噪信号保存的文件名"="AI114.csv" ("name or relative path"), "sym"=w1189, "数组中的数据（输入）"=w1194, "lev"=w1190) -> ("字符串（输出）"=→"特征值15":string, "特征值（输出）"=→"AI14特征值":dbl[][], "去噪后波形图"=→"AI14去噪后波形图":dbl[][])  [unwired: 4 in]
                          }
                          frame #1 {
                            n611 = local read "特征值15"() -> (w1199:string)
                            n612 = Concatenate Strings("insert into sensor15(value1,value2,value3,value4,value5,value6,value7,value8) values(" ("Command Text"), w1199, ");") -> (w1200:string)
                            n613 = call "SQL Execute.vi"("error in (no error)"=w1197, "Return Data (T)"=FALSE, "Command Text"=w1200, "ADODB._Connection In"=w1198) -> ()  [unwired: 4 in, 4 out]
                          }
                        }
                      }
                    }
                  }
                  frame #16 {
                    n614 = local read "AI15"() -> (w1208:bool)
                    n615 = case shown="真" w1208 {
                      tunnel: w1207 -> [_ w1212]
                      tunnel: w1206 -> [_ w1211]
                      tunnel: w1205 -> [_ w1210]
                      tunnel: w1204 -> [_ w1209]
                      frame False {
                      }
                      frame True {
                        n616 = flat-sequence {
                          tunnel: w1210 -> [w1214]
                          tunnel: w1209 -> [w1213]
                          tunnel: w1212 -> [w1222]
                          tunnel: w1211 -> [w1221]
                          frame #0 {
                            n617 = local read "输出数组16"() -> (w1220:dbl[])
                            n618 = call "数据处理2.vi"("原始数据文件名"="AI15.csv" ("name or relative path"), "去噪信号保存的文件名"="AI115.csv" ("name or relative path"), "sym"=w1213, "数组中的数据（输入）"=w1220, "lev"=w1214) -> ("字符串（输出）"=→"特征值16":string, "特征值（输出）"=→"AI15特征值":dbl[][], "去噪后波形图"=→"AI15去噪后波形图":dbl[][])  [unwired: 4 in]
                          }
                          frame #1 {
                            n619 = local read "特征值16"() -> (w1223:string)
                            n620 = Concatenate Strings("insert into sensor16(value1,value2,value3,value4,value5,value6,value7,value8) values(" ("Command Text"), w1223, ");") -> (w1224:string)
                            n621 = call "SQL Execute.vi"("error in (no error)"=w1221, "Return Data (T)"=FALSE, "Command Text"=w1224, "ADODB._Connection In"=w1222) -> ()  [unwired: 4 in, 4 out]
                          }
                        }
                      }
                    }
                  }
                }
              }
            }
          }
          frame #3 {
            # "复位"
            n622 = invoke on="输出数组5" class="Arr (严格)" method="Reinit To Default"() -> ()  [unwired: 3 in, 3 out]
            n623 = invoke on="输出数组2" class="Arr (严格)" method="Reinit To Default"() -> ()  [unwired: 3 in, 3 out]
            n624 = invoke on="输出数组3" class="Arr (严格)" method="Reinit To Default"() -> ()  [unwired: 3 in, 3 out]
            n625 = invoke on="输出数组4" class="Arr (严格)" method="Reinit To Default"() -> ()  [unwired: 3 in, 3 out]
            n626 = invoke on="输出数组6" class="Arr (严格)" method="Reinit To Default"() -> ()  [unwired: 3 in, 3 out]
            n627 = invoke on="输出数组8" class="Arr (严格)" method="Reinit To Default"() -> ()  [unwired: 3 in, 3 out]
            n628 = invoke on="输出数组7" class="Arr (严格)" method="Reinit To Default"() -> ()  [unwired: 3 in, 3 out]
            n629 = invoke on="输出数组1" class="Arr (严格)" method="Reinit To Default"() -> ()  [unwired: 3 in, 3 out]
            n630 = invoke on="输出数组9" class="Arr (严格)" method="Reinit To Default"() -> ()  [unwired: 3 in, 3 out]
            n631 = invoke on="输出数组10" class="Arr (严格)" method="Reinit To Default"() -> ()  [unwired: 3 in, 3 out]
            n632 = invoke on="输出数组12" class="Arr (严格)" method="Reinit To Default"() -> ()  [unwired: 3 in, 3 out]
            n633 = invoke on="输出数组11" class="Arr (严格)" method="Reinit To Default"() -> ()  [unwired: 3 in, 3 out]
            n634 = invoke on="输出数组13" class="Arr (严格)" method="Reinit To Default"() -> ()  [unwired: 3 in, 3 out]
            n635 = invoke on="输出数组14" class="Arr (严格)" method="Reinit To Default"() -> ()  [unwired: 3 in, 3 out]
            n636 = invoke on="输出数组15" class="Arr (严格)" method="Reinit To Default"() -> ()  [unwired: 3 in, 3 out]
            n637 = invoke on="输出数组16" class="Arr (严格)" method="Reinit To Default"() -> ()  [unwired: 3 in, 3 out]
          }
          frame #4 {
            # "延时"
            n638 = local read "延时"() -> (w1228:bool)
            n639 = case shown="真" w1228 {
              frame False {
              }
              frame True {
                n640 = Multiply(x="间隔时间", y=60000) -> (x*y=w1230:i32)
                n641 = Wait (ms)(milliseconds to wait=w1230) -> ()  [unwired: 1 out]
              }
            }
          }
        }
        n642 = call "StopRead.vi"("错误输入（无错误）"=w241, "DevIndex"=w242) -> ("错误输出"=w267:errorcluster, "DevIndex Output"=w268:i32)  [unwired: 8 in]
        n643 = call "SetSoftTrig.vi"("错误输入（无错误）"=w267, "Trig"=u8 0, "DevIndex"=w268) -> ("错误输出"=w272:errorcluster, "DevIndex Output"=w271:i32)  [unwired: 7 in]
        n644 = call "ClearBufs.vi"("错误输入（无错误）"=w272, "DevIndex"=w271) -> ("错误输出"=w270:errorcluster, "DevIndex Output"=w269:i32)  [unwired: 8 in]
        n645 = call "CloseDevice.vi"("错误输入（无错误）"=w270, "DevIndex"=w269) -> ("错误输出"=w202:errorcluster)  [unwired: 8 in, 1 out]
        n646 = local write "采集卡状态"(w202) -> ()
      }
    }
  }
  n647 = while {
    stop <- FALSE stop-if-true
    # "初始化"
    n648 = event shown="[1] \"初始化\": 鼠标释放" {
      selector: _ -> [_ _]
      dyn-events: _ -> [_ _]
      timeout: _ -> [_ _]
      event Timeout {
        n649 = event-data() -> ()  [unwired: 1 in, 3 out]
      }
      event "初始化": Mouse Up {
        n650 = event-data() -> ()  [unwired: 1 in, 8 out]
        n651 = stacked-sequence {
          frame #0 {
            n652 = invoke on="当前组波形" class="WFGraph (严格)" method="Reinit To Default"() -> ()  [unwired: 3 in, 3 out]
            n653 = invoke on="延时" class="Bool (严格)" method="Reinit To Default"() -> ()  [unwired: 3 in, 3 out]
            n654 = invoke on="开始" class="Bool (严格)" method="Reinit To Default"() -> ()  [unwired: 3 in, 3 out]
            n655 = invoke on="数据库" class="Bool (严格)" method="Reinit To Default"() -> ()  [unwired: 3 in, 3 out]
            n656 = invoke on="通道选择" class="Arr (严格)" method="Reinit To Default"() -> ()  [unwired: 3 in, 3 out]
            n657 = invoke on="AI 1 波形" class="WFGraph (strict)" method="Reinit To Default"() -> ()  [unwired: 3 in, 3 out]
            n658 = invoke on="AI 2 波形" class="WFGraph (strict)" method="Reinit To Default"() -> ()  [unwired: 3 in, 3 out]
            n659 = invoke on="AI 3 波形" class="WFGraph (strict)" method="Reinit To Default"() -> ()  [unwired: 3 in, 3 out]
            n660 = invoke on="AI 4 波形" class="WFGraph (strict)" method="Reinit To Default"() -> ()  [unwired: 3 in, 3 out]
            n661 = invoke on="AI 5 波形" class="WFGraph (strict)" method="Reinit To Default"() -> ()  [unwired: 3 in, 3 out]
            n662 = invoke on="AI 6 波形" class="WFGraph (strict)" method="Reinit To Default"() -> ()  [unwired: 3 in, 3 out]
            n663 = invoke on="AI 7 波形" class="WFGraph (strict)" method="Reinit To Default"() -> ()  [unwired: 3 in, 3 out]
            n664 = invoke on="数据处理" class="Bool (严格)" method="Reinit To Default"() -> ()  [unwired: 3 in, 3 out]
            n665 = invoke on="上传到数据库" class="Bool (strict)" method="Reinit To Default"() -> ()  [unwired: 3 in, 3 out]
            n666 = invoke on="查看单传感器采集的数据" class="Bool" method="Reinit To Default"() -> ()  [unwired: 3 in, 3 out]
            n667 = invoke on="创建特征值数据表" class="Bool" method="Reinit To Default"() -> ()  [unwired: 3 in, 3 out]
            n668 = invoke on="AI 8 波形" class="WFGraph (strict)" method="Reinit To Default"() -> ()  [unwired: 3 in, 3 out]
            n669 = invoke on="AI 9 波形" class="WFGraph (strict)" method="Reinit To Default"() -> ()  [unwired: 3 in, 3 out]
            n670 = invoke on="AI 10 波形" class="WFGraph (strict)" method="Reinit To Default"() -> ()  [unwired: 3 in, 3 out]
            n671 = invoke on="AI 11 波形" class="WFGraph (strict)" method="Reinit To Default"() -> ()  [unwired: 3 in, 3 out]
            n672 = invoke on="AI 12 波形" class="WFGraph (strict)" method="Reinit To Default"() -> ()  [unwired: 3 in, 3 out]
            n673 = invoke on="AI 13 波形" class="WFGraph (strict)" method="Reinit To Default"() -> ()  [unwired: 3 in, 3 out]
            n674 = invoke on="AI 14 波形" class="WFGraph (strict)" method="Reinit To Default"() -> ()  [unwired: 3 in, 3 out]
            n675 = invoke on="AI 15 波形" class="WFGraph (strict)" method="Reinit To Default"() -> ()  [unwired: 3 in, 3 out]
            n676 = invoke on="AI 1 size(s)" class="DigNum (strict)" method="Reinit To Default"() -> ()  [unwired: 3 in, 3 out]
            n677 = invoke on="AI 5 size(s)" class="DigNum (strict)" method="Reinit To Default"() -> ()  [unwired: 3 in, 3 out]
            n678 = invoke on="AI 6 size(s)" class="DigNum (strict)" method="Reinit To Default"() -> ()  [unwired: 3 in, 3 out]
            n679 = invoke on="AI 7 size(s)" class="DigNum (strict)" method="Reinit To Default"() -> ()  [unwired: 3 in, 3 out]
            n680 = invoke on="AI 0 size(s)" class="DigNum (严格)" method="Reinit To Default"() -> ()  [unwired: 3 in, 3 out]
            n681 = invoke on="AI 2 size(s)" class="DigNum (strict)" method="Reinit To Default"() -> ()  [unwired: 3 in, 3 out]
            n682 = invoke on="AI 3 size(s)" class="DigNum (strict)" method="Reinit To Default"() -> ()  [unwired: 3 in, 3 out]
            n683 = invoke on="AI 4 size(s)" class="DigNum (strict)" method="Reinit To Default"() -> ()  [unwired: 3 in, 3 out]
            n684 = invoke on="关闭" class="Bool (严格)" method="Reinit To Default"() -> ()  [unwired: 3 in, 3 out]
            n685 = invoke on="创建原始数据表" class="Bool" method="Reinit To Default"() -> ()  [unwired: 3 in, 3 out]
            n686 = invoke on="传感器数据查询" class="Bool" method="Reinit To Default"() -> ()  [unwired: 3 in, 3 out]
            n687 = invoke on="健康值查询" class="Bool" method="Reinit To Default"() -> ()  [unwired: 3 in, 3 out]
            n688 = invoke on="AI 8 size(s)" class="DigNum (strict)" method="Reinit To Default"() -> ()  [unwired: 3 in, 3 out]
            n689 = invoke on="AI 9 size(s)" class="DigNum (strict)" method="Reinit To Default"() -> ()  [unwired: 3 in, 3 out]
            n690 = invoke on="AI 10 size(s)" class="DigNum (strict)" method="Reinit To Default"() -> ()  [unwired: 3 in, 3 out]
            n691 = invoke on="AI 11 size(s)" class="DigNum (strict)" method="Reinit To Default"() -> ()  [unwired: 3 in, 3 out]
            n692 = invoke on="AI 12 size(s)" class="DigNum (strict)" method="Reinit To Default"() -> ()  [unwired: 3 in, 3 out]
            n693 = invoke on="AI 13 size(s)" class="DigNum (strict)" method="Reinit To Default"() -> ()  [unwired: 3 in, 3 out]
            n694 = invoke on="AI 14 size(s)" class="DigNum (strict)" method="Reinit To Default"() -> ()  [unwired: 3 in, 3 out]
            n695 = invoke on="AI 15 size(s)" class="DigNum (strict)" method="Reinit To Default"() -> ()  [unwired: 3 in, 3 out]
            n696 = invoke on="暂停" class="Bool" method="Reinit To Default"() -> ()  [unwired: 3 in, 3 out]
            n697 = invoke on="查看去噪后波形" class="Bool" method="Reinit To Default"() -> ()  [unwired: 3 in, 3 out]
            n698 = invoke on="查看当前数据波形" class="Bool" method="Reinit To Default"() -> ()  [unwired: 3 in, 3 out]
            n699 = invoke on="查看当前特征值" class="Bool" method="Reinit To Default"() -> ()  [unwired: 3 in, 3 out]
            n700 = invoke on="AI0去噪后波形图" class="WFGraph (strict)" method="Reinit To Default"() -> ()  [unwired: 3 in, 3 out]
            n701 = invoke on="AI1去噪后波形图" class="WFGraph (strict)" method="Reinit To Default"() -> ()  [unwired: 3 in, 3 out]
            n702 = invoke on="AI2去噪后波形图" class="WFGraph (strict)" method="Reinit To Default"() -> ()  [unwired: 3 in, 3 out]
            n703 = invoke on="AI3去噪后波形图" class="WFGraph (strict)" method="Reinit To Default"() -> ()  [unwired: 3 in, 3 out]
            n704 = invoke on="AI4去噪后波形图" class="WFGraph (strict)" method="Reinit To Default"() -> ()  [unwired: 3 in, 3 out]
            n705 = invoke on="AI5去噪后波形图" class="WFGraph (strict)" method="Reinit To Default"() -> ()  [unwired: 3 in, 3 out]
            n706 = invoke on="AI6去噪后波形图" class="WFGraph (strict)" method="Reinit To Default"() -> ()  [unwired: 3 in, 3 out]
            n707 = invoke on="AI7去噪后波形图" class="WFGraph (strict)" method="Reinit To Default"() -> ()  [unwired: 3 in, 3 out]
            n708 = invoke on="主页按钮" class="Bool" method="Reinit To Default"() -> ()  [unwired: 3 in, 3 out]
            n709 = invoke on="主页按钮 2" class="Bool" method="Reinit To Default"() -> ()  [unwired: 3 in, 3 out]
            n710 = invoke on="主页按钮 3" class="Bool" method="Reinit To Default"() -> ()  [unwired: 3 in, 3 out]
            n711 = invoke on="AI8去噪后波形图" class="WFGraph (strict)" method="Reinit To Default"() -> ()  [unwired: 3 in, 3 out]
            n712 = invoke on="AI9去噪后波形图" class="WFGraph (strict)" method="Reinit To Default"() -> ()  [unwired: 3 in, 3 out]
            n713 = invoke on="AI10去噪后波形图" class="WFGraph (strict)" method="Reinit To Default"() -> ()  [unwired: 3 in, 3 out]
            n714 = invoke on="AI11去噪后波形图" class="WFGraph (strict)" method="Reinit To Default"() -> ()  [unwired: 3 in, 3 out]
            n715 = invoke on="AI2去噪后波形图" class="WFGraph (strict)" method="Reinit To Default"() -> ()  [unwired: 3 in, 3 out]
            n716 = invoke on="AI13去噪后波形图" class="WFGraph (strict)" method="Reinit To Default"() -> ()  [unwired: 3 in, 3 out]
            n717 = invoke on="AI14去噪后波形图" class="WFGraph (strict)" method="Reinit To Default"() -> ()  [unwired: 3 in, 3 out]
            n718 = invoke on="AI15去噪后波形图" class="WFGraph (strict)" method="Reinit To Default"() -> ()  [unwired: 3 in, 3 out]
            n719 = invoke on="主页按钮 4" class="Bool" method="Reinit To Default"() -> ()  [unwired: 3 in, 3 out]
            n720 = invoke on="主页按钮 5" class="Bool" method="Reinit To Default"() -> ()  [unwired: 3 in, 3 out]
            n721 = invoke on="主页按钮 6" class="Bool" method="Reinit To Default"() -> ()  [unwired: 3 in, 3 out]
            n722 = invoke on="AI0特征值" class="Arr (strict)" method="Reinit To Default"() -> ()  [unwired: 3 in, 3 out]
            n723 = invoke on="AI1特征值" class="Arr (strict)" method="Reinit To Default"() -> ()  [unwired: 3 in, 3 out]
            n724 = invoke on="AI2特征值" class="Arr (strict)" method="Reinit To Default"() -> ()  [unwired: 3 in, 3 out]
            n725 = invoke on="AI3特征值" class="Arr (strict)" method="Reinit To Default"() -> ()  [unwired: 3 in, 3 out]
            n726 = invoke on="AI4特征值" class="Arr (strict)" method="Reinit To Default"() -> ()  [unwired: 3 in, 3 out]
            n727 = invoke on="AI5特征值" class="Arr (strict)" method="Reinit To Default"() -> ()  [unwired: 3 in, 3 out]
            n728 = invoke on="AI6特征值" class="Arr (strict)" method="Reinit To Default"() -> ()  [unwired: 3 in, 3 out]
            n729 = invoke on="AI7特征值" class="Arr (strict)" method="Reinit To Default"() -> ()  [unwired: 3 in, 3 out]
            n730 = invoke on="主页按钮 7" class="Bool" method="Reinit To Default"() -> ()  [unwired: 3 in, 3 out]
            n731 = invoke on="主页按钮 8" class="Bool" method="Reinit To Default"() -> ()  [unwired: 3 in, 3 out]
            n732 = invoke on="主页按钮 9" class="Bool" method="Reinit To Default"() -> ()  [unwired: 3 in, 3 out]
            n733 = invoke on="AI8特征值" class="Arr (strict)" method="Reinit To Default"() -> ()  [unwired: 3 in, 3 out]
            n734 = invoke on="AI9特征值" class="Arr (strict)" method="Reinit To Default"() -> ()  [unwired: 3 in, 3 out]
            n735 = invoke on="AI10特征值" class="Arr (strict)" method="Reinit To Default"() -> ()  [unwired: 3 in, 3 out]
            n736 = invoke on="AI11特征值" class="Arr (strict)" method="Reinit To Default"() -> ()  [unwired: 3 in, 3 out]
            n737 = invoke on="AI12特征值" class="Arr (strict)" method="Reinit To Default"() -> ()  [unwired: 3 in, 3 out]
            n738 = invoke on="AI13特征值" class="Arr (strict)" method="Reinit To Default"() -> ()  [unwired: 3 in, 3 out]
            n739 = invoke on="AI14特征值" class="Arr (strict)" method="Reinit To Default"() -> ()  [unwired: 3 in, 3 out]
            n740 = invoke on="AI15特征值" class="Arr (strict)" method="Reinit To Default"() -> ()  [unwired: 3 in, 3 out]
            n741 = invoke on="状态提示" class="Str" method="Reinit To Default"() -> ()  [unwired: 3 in, 3 out]
            n742 = invoke on="sym" class="Str" method="Reinit To Default"() -> ()  [unwired: 3 in, 3 out]
            n743 = invoke on="健康值查询结果" class="Tbl (严格)" method="Reinit To Default"() -> ()  [unwired: 3 in, 3 out]
            n744 = invoke on="过程提示" class="Str" method="Reinit To Default"() -> ()  [unwired: 3 in, 3 out]
            n745 = invoke on="查询数据" class="Tbl (strict)" method="Reinit To Default"() -> ()  [unwired: 3 in, 3 out]
            n746 = invoke on="全部数据" class="Tbl (strict)" method="Reinit To Default"() -> ()  [unwired: 3 in, 3 out]
            n747 = invoke on="当前时间" class="AbsTime (严格)" method="Reinit To Default"() -> ()  [unwired: 3 in, 3 out]
            n748 = invoke on="数据库状态" class="Clust (严格)" method="Reinit To Default"() -> ()  [unwired: 3 in, 3 out]
            n749 = invoke on="采集卡状态" class="Clust (严格)" method="Reinit To Default"() -> ()  [unwired: 3 in, 3 out]
            n750 = invoke on="lev" class="DigNum (严格)" method="Reinit To Default"() -> ()  [unwired: 3 in, 3 out]
            n751 = invoke on="采样率" class="DigNum (严格)" method="Reinit To Default"() -> ()  [unwired: 3 in, 3 out]
            n752 = invoke on="数据处理及上传控制" class="DigNum (严格)" method="Reinit To Default"() -> ()  [unwired: 3 in, 3 out]
          }
          frame #1 {
            n753 = One Button Dialog(message="初始化完成！！！" ("消息")) -> ()  [unwired: 1 in, 1 out]
          }
        }
      }
    }
  }
  n754 = while {
    stop <- FALSE stop-if-true
    # "选项卡跳转控制"
    n755 = event shown="[9] \"搜索按钮\": 鼠标释放" {
      selector: _ -> [_ _ _ _ _ _ _ _ _ _]
      dyn-events: _ -> [_ _ _ _ _ _ _ _ _ _]
      timeout: _ -> [_ _ _ _ _ _ _ _ _ _]
      event Timeout {
        n756 = event-data() -> ()  [unwired: 1 in, 3 out]
      }
      event "传感器数据查询": Mouse Up {
        n757 = event-data() -> ()  [unwired: 1 in, 8 out]
        n758 = property on="历史查询选项卡" class="TabCtl (严格)"("Value"=enum32{"原始数据查询", "健康值查询"}."原始数据查询" ("历史查询选项卡")) -> ()  [unwired: 2 in, 2 out]
      }
      event "主页按钮", "主页按钮 2", "主页按钮 3", "主页按钮 4", "主页按钮 5", "主页按钮 6", "主页按钮 7", "主页按钮 8", "主页按钮 9": Mouse Up {
        n759 = event-data() -> ()  [unwired: 1 in, 8 out]
        n760 = property on="主选项卡" class="TabCtl (严格)"("Value"=T1."端口设置" ("主选项卡")) -> ()  [unwired: 2 in, 2 out]
      }
      event "健康值查询": Mouse Up {
        n761 = event-data() -> ()  [unwired: 1 in, 8 out]
        n762 = property on="历史查询选项卡" class="TabCtl (严格)"("Value"=enum32{"原始数据查询", "健康值查询"}."健康值查询" ("历史查询选项卡")) -> ()  [unwired: 2 in, 2 out]
      }
      event "查看去噪后波形": Mouse Up {
        n763 = event-data() -> ()  [unwired: 1 in, 8 out]
        n764 = property on="主选项卡" class="TabCtl (严格)"("Value"=T1."去噪后的波形" ("主选项卡")) -> ()  [unwired: 2 in, 2 out]
      }
      event "查看当前数据波形": Mouse Up {
        n765 = event-data() -> ()  [unwired: 1 in, 8 out]
        n766 = property on="主选项卡" class="TabCtl (严格)"("Value"=T1."原始数据波形" ("主选项卡")) -> ()  [unwired: 2 in, 2 out]
      }
      event "查看当前特征值": Mouse Up {
        n767 = event-data() -> ()  [unwired: 1 in, 8 out]
        n768 = property on="主选项卡" class="TabCtl (严格)"("Value"=T1."特征值数据" ("主选项卡")) -> ()  [unwired: 2 in, 2 out]
      }
      event "历史查询": Mouse Up {
        n769 = event-data() -> ()  [unwired: 1 in, 8 out]
        n770 = property on="主选项卡" class="TabCtl (严格)"("Value"=T1."历史查询" ("主选项卡")) -> ()  [unwired: 2 in, 2 out]
      }
      event "查看单传感器采集的数据": Mouse Up {
        n771 = event-data() -> ()  [unwired: 1 in, 8 out]
        n772 = property on="主选项卡" class="TabCtl (严格)"("Value"=T1."单传感器测试" ("主选项卡")) -> ()  [unwired: 2 in, 2 out]
      }
      event "搜索按钮": Mouse Up {
        n773 = event-data() -> ()  [unwired: 1 in, 8 out]
        n774 = property on="主选项卡" class="TabCtl (严格)"("Value"=T1."传感器数据" ("主选项卡")) -> ()  [unwired: 2 in, 2 out]
      }
    }
  }
  n775 = while {
    stop <- w1244 stop-if-true
    # "功能状态监测"
    n776 = Get Date/Time In Seconds() -> (seconds since 1Jan1904=→"当前时间":timestamp)
    n777 = local read "关闭"() -> (w1244:bool)
    n778 = Quit LabVIEW(quit? (T)=w1244) -> ()
    "数据处理 2" <- "数据处理"
  }
  "数据处理及上传控制" <- 0
